vi "Steuerprogramm-04-02-17.vi"() -> ()   [LabVIEW 2010]
uses:
  Emil/Licor-Steuerung/HAGAR V/Licor-Steuerung/display/GUI_Cluster_sdv.ctl
  Emil/Licor-Steuerung/HAGAR V/Licor-Steuerung/display/GUI_Cluster_Parameter.ctl
  Emil/Licor-Steuerung/HAGAR V/Licor-Steuerung/control/Licor-Commands.ctl
  Emil/Licor-Steuerung/HAGAR V/Licor-Steuerung/control/Licor-Parameter.ctl
  Emil/Licor-Steuerung/LicorLI7000/conventions/Licor-Source.ctl
  Emil/Licor-Steuerung/HAGAR V/Licor-Steuerung/control/Licor-Pump.ctl
  Emil/Licor-Steuerung/HAGAR V/Licor-Steuerung/display/GUI_Cluster_Graph.ctl
  Emil/Licor-Steuerung/HAGAR V/Licor-Steuerung/control/Licor-Sequences.ctl
  <vilib>/rvi/interface/nirviMethod/nirviMethod.xnode
  C:/Users/HAGAR-IV/Desktop/Zeugs/markus/version feb 2012/FPGA Bitfiles/pertrasgcfpga2_FPGATarget_FPGA-Programm-01_A75D3647.lvbitx
  C:/Users/HAGAR-IV/Desktop/Zeugs/Johnny/pertrasgc fpga/FPGA-Programm-01-17.vi
  <vilib>/rvi/interface/common/niFpgaNodeNameForErrorReporting.ctl
  <vilib>/rvi/errors/niLvFpgaWhatHappensToTopLevelVI.ctl
  <vilib>/rvi/interface/nirviReadWriteControl/nirviReadWriteControl.xnode
  <vilib>/rvi/interface/nirviCloseFPGA/nirviCloseFPGA.xnode
  GVZwangs.vi
  GVProbenvol.vi
  GVZeitenZyklen.vi
  GVECDs.vi
  GVMethodenwechsel.vi
  GVTrapsMachs.vi
  GVHK1Hz.vi
  GVAIs.vi
  gvbooleschRT.vi
  GVMetavariablen.vi
  GVVentilposition.vi
  GVHorstSP.vi
  GVMWHorst.vi
  GVHeizenLH.vi
  <vilib>/Utility/error.llb/Error Cluster From Error Code.vi
  <vilib>/rvi/errors/niLvFpgaAdjustHostInterfaceError.vi
  GVaktuelleTDMS.vi
  Emil/Licor-Steuerung/HAGAR V/Licor-Steuerung/control/Emulate Licor output GV.vi
  GVChroms.vi
  GVZwangsMPV.vi
  <vilib>/FPGAPlugInAG/cRIO-9114/niLvFpga_Close_cRIO-9114.vi
  NiFpgaLv.dll
  Emil/Licor-Steuerung/HAGAR V/Licor-Steuerung/Licor-Steuerung.lvlib
  Emil/Licor-Steuerung/LicorLI7000/LicorLI7000.lvlib
panel:
  in  "Handbetrieb":bool
  in  "Methode speichern":bool
  out "ZyklusNummernGesamt":i32[](array[numeric])
  in  "veränderte Methode benutzen":bool
  in  "Methode verändern":bool
  out "ZyklusNummern":i32[](array[numeric])
  out "Big Ben, Methodenzeit, Zykluszeit0, Zykluszeit1, Zykluszeit2A, Zykluszeit2B":i32[](array[numeric])
  in  "global stop RT":bool
  in  "Methode":i32(ring) items=["Bedingsmethode", "Startmethode", "Meßmodus", "Shut-up-Methode", "Test", "HAG2 1/2", "Startmethode", "HAG2 1/2 Aufwärmen"]
  in  "Registerkarte":T1(tab)
  out "SHOK?":bool[](array[boolean])
  out "schnelle Heizungen":string[](array[string])
  out "schnelle Heizungen":dbl[](array[numeric])
  out "HorstOK?":bool[](array[boolean])
  out "AIs3OK?":bool[](array[boolean])
  out "AIs1OK?":bool[](array[boolean])
  out "AIs1":dbl[](array[numeric])
  out "AIs1":string[](array[string])
  out "AIs2":string[](array[string])
  out "AIs3":string[](array[string])
  out "AIs2":dbl[](array[numeric])
  out "AIs3":dbl[](array[numeric])
  out "Metavariablen":string[](array[string])
  out "Metavariablen":dbl[](array[numeric])
  out "MWHorst":dbl[](array[numeric])
  out "HorstRegler":string[](array[string])
  out "AIs2OK?":bool[](array[boolean])
  out "Ventilposition":i32=1 min=1 max=6 step=1
  out "MVOK?":bool[](array[boolean])
  in  "Color Box":u32(colorbox)
  out "Numeric":dbl
  out "Housekeeping1":cluster{dbl[], dbl[]}(graph)
  in  "Zeitachse1":i32(ring)=1 items=["Zykluszeit [s] Mod0", "Zykluszeit [s] Mod1", "Zykluszeit [s] Mod2A", "Zykluszeit [s] Mod2B"]
  in  "dargestellte Größe 1":i32(ring)=1 items=["T1-Trap1", "T1-Trap2", "T1-StirlingKühlkopf", "T1-PreCol1", "T1-PreCol2", "T1-MainCol1a", "T1-MainCol1b", "T1-MainCol2a", "T1-MainCol2b", "T1-Bronkhorst1a", "T1-Bronkhorst1b", "T1-Bronkhorst2a", "T1-Bronkhorst2b", "T1-2Pos1B", "T1-Spare9", "T1-2Pos1A", "T1-Spare10", "T1-TurboPump", "T1-StirlingPlatine", "T1-Spare5", "T1-Spare6", "T1-Spare7", "T1-Spare8", "F1-MFM1", "F1-MFM0D [mL]", "P1-MethaneHP", "P1-MethaneLP", "P1-Vacuum", "TurboSpeed", "I1-MS-AC", "I1-Trap1", "I1-Trap2", "T2-ECD1a", "T2-ECD1b", "T2-ECD2a", "T2-ECD2b", "T2-Col1a", "T2-Col1b", "T2-Col2a", "T2-Col2b", "T2-Spare1", "T2-Spare2", "T2-Oven_a", "T2-Oven_b", "T2-Spare3", "T2-Spare4", "T2-Spare5", "F2-MFM0", "F2-MFM2A", "F2-MFM2B", "P2-N2O_HP", "P2-N2O_LP", "P2-CO2_HP", "P2-CO2_LP", "AI-Spare1", "FL-MFM1000mL", "AI-Spare3", "AI-Spare4", "StirlingAlarm", "StirlingEmerg.", "AI-Spare7", "AI-Spare8", "AI-Spare9", "FL-MFM30mL", "T0-DC/DC5", "I0-24V_M0", "I0-48V_M1", "I0-24V_M1", "I0-28V_M2", "T0-Spare3", "T0-Spare2", "T0-Spare4", "T0-DC/DC7", "I0-20V_Laptop", "I0-28V_M1", "I0-24V_M2", "I0-12V_Licor", "T0-Spare1", "T0-Drier", "T0-Spare5", "F0-MFM0A [L]", "TL-Licor_a", "P0-Span-HP", "P0-spare1", "P0-Stickstoff-LP", "P0-Helium-LP", "P0-Cal-HP", "P0-P9Tavco[bar]", "F0-MFM0B [L]", "TL-Licor_b", "P0-Span-LP", "P0-spare2", "P0-Stickstoff-HP", "P0-Helium-HP", "P0-Cal-LP", "F0-MFM3", "TemperaturTrap1[°C]", "TemperaturTrap2[°C]", "TemperaturPreMach1[°C]", "TemperaturPreMach2[°C]", "TemperaturMainMach1[°C]", "TemperaturMainMach2[°C]", "PrC0", "PrC0-Licor", "PrC1-Säule2", "PrC1-Säule1", "MFC1-Sample", "MFC1-Methan", "PrC1-BackFlush1", "PrC1-BackFlush2", "MFC2A", "MFC2B", "MFC2C", "PrC2A", "MFC2D", "MFC2E", "PrC2B"]
  out "Housekeeping2":cluster{dbl[], dbl[]}(graph)
  in  "Zeitachse2":i32(ring)=1 items=["Zykluszeit [s] Mod0", "Zykluszeit [s] Mod1", "Zykluszeit [s] Mod2A", "Zykluszeit [s] Mod2B"]
  in  "dargestellte Größe 2":i32(ring)=1 items=["T1-Trap1", "T1-Trap2", "T1-StirlingKühlkopf", "T1-PreCol1", "T1-PreCol2", "T1-MainCol1a", "T1-MainCol1b", "T1-MainCol2a", "T1-MainCol2b", "T1-Bronkhorst1a", "T1-Bronkhorst1b", "T1-Bronkhorst2a", "T1-Bronkhorst2b", "T1-2Pos1B", "T1-Spare9", "T1-2Pos1A", "T1-Spare10", "T1-TurboPump", "T1-StirlingPlatine", "T1-Spare5", "T1-Spare6", "T1-Spare7", "T1-Spare8", "F1-MFM1", "F1-MFM0D [mL]", "P1-MethaneHP", "P1-MethaneLP", "P1-Vacuum", "TurboSpeed", "I1-MS-AC", "I1-Trap1", "I1-Trap2", "T2-ECD1a", "T2-ECD1b", "T2-ECD2a", "T2-ECD2b", "T2-Col1a", "T2-Col1b", "T2-Col2a", "T2-Col2b", "T2-Spare1", "T2-Spare2", "T2-Oven_a", "T2-Oven_b", "T2-Spare3", "T2-Spare4", "T2-Spare5", "F2-MFM0", "F2-MFM2A", "F2-MFM2B", "P2-N2O_HP", "P2-N2O_LP", "P2-CO2_HP", "P2-CO2_LP", "AI-Spare1", "FL-MFM1000mL", "AI-Spare3", "AI-Spare4", "StirlingAlarm", "StirlingEmerg.", "AI-Spare7", "AI-Spare8", "AI-Spare9", "FL-MFM30mL", "T0-DC/DC5", "I0-24V_M0", "I0-48V_M1", "I0-24V_M1", "I0-28V_M2", "T0-Spare3", "T0-Spare2", "T0-Spare4", "T0-DC/DC7", "I0-20V_Laptop", "I0-28V_M1", "I0-24V_M2", "I0-12V_Licor", "T0-Spare1", "T0-Drier", "T0-Spare5", "F0-MFM0A [L]", "TL-Licor_a", "P0-Span-HP", "P0-spare1", "P0-Stickstoff-LP", "P0-Helium-LP", "P0-Cal-HP", "P0-P9Tavco[bar]", "F0-MFM0B [L]", "TL-Licor_b", "P0-Span-LP", "P0-spare2", "P0-Stickstoff-HP", "P0-Helium-HP", "P0-Cal-LP", "F0-MFM3", "TemperaturTrap1[°C]", "TemperaturTrap2[°C]", "TemperaturPreMach1[°C]", "TemperaturPreMach2[°C]", "TemperaturMainMach1[°C]", "TemperaturMainMach2[°C]", "PrC0", "PrC0-Licor", "PrC1-Säule2", "PrC1-Säule1", "MFC1-Sample", "MFC1-Methan", "PrC1-BackFlush1", "PrC1-BackFlush2", "MFC2A", "MFC2B", "MFC2C", "PrC2A", "MFC2D", "MFC2E", "PrC2B"]
  out "Detektor 2":cluster{dbl[], dbl[]}[](graph)
  in  "Detektor":i32(ring) items=["ECD1", "ECD2"]
  in  "HK1YMin":dbl
  in  "HK1YMax":dbl=100.0
  in  "HK2YMin":dbl
  in  "HK2YMax":dbl=100.0
  in  "DetYMin":dbl
  in  "DetYMax":dbl=100.0
  out "schnelleAnzeige":cluster{dbl[], dbl[]}(graph)
  in  "TafelWischen!":bool
  in  "dargestellte Größe 3":i32(ring)=1 items=["TemperaturTrap1[°C]", "TemperaturTrap2[°C]", "TemperaturPreMach1[°C]", "TemperaturPreMach2[°C]", "TemperaturMainMach1[°C]", "TemperaturMainMach2[°C]", "PrC0", "PrC0-Licor", "PrC1-Säule2", "PrC1-Säule1", "MFC1-Sample", "MFC1-Methan", "PrC1-BackFlush1", "PrC1-BackFlush2", "MFC2A", "MFC2B", "MFC2C", "PrC2A", "MFC2D", "MFC2E", "PrC2B"]
  in  "An/Aus":bool
  in  "Registerkarte 2":T2(tab)
  in  "GUI_Cluster_Graph":T3={"time (global)"=0.0, "command queue"=[], "Rohdaten"=[], "Graph"={"X"=[], "Y"=[]}, "Manuelle Steuerung"={"Sequenz"=enum."test", "Manuelle Steuerung An/Aus"=FALSE}, "Sequenz out"={"sequence"=enum."WAIT", "Zeitpunkt next"=0.0, "delta t"=0.0}} caption="Cluster" {"Sequenz out"."Zeitpunkt next" format="%<%H:%M:%S%3u>T"; "time (global)" format="%<%H:%M:%S%3u\n%m/%d/%y>T"}
  in  "GUI_Cluster_Parameter":T5={"warmup (sequence)"=[{"time"=60, "Enum"=enum."wait"}], "calibrate S (sequence)"=[{"time"=60, "Enum"=enum."wait"}, {"time"=2, "Enum"=enum."getCalibrationParameter"}, {"time"=8, "Enum"=enum."calibration-S-CO2"}, {"time"=2, "Enum"=enum."getCalibrationParameter"}], "calibrate Z (sequence)"=[{"time"=60, "Enum"=enum."wait"}, {"time"=2, "Enum"=enum."getCalibrationParameter"}, {"time"=8, "Enum"=enum."calibration-Z-H2O"}, {"time"=2, "Enum"=enum."getCalibrationParameter"}, {"time"=8, "Enum"=enum."calibration-Z-CO2"}, {"time"=2, "Enum"=enum."getCalibrationParameter"}], "initialize (sequence)"=[{"time"=30, "Enum"=enum."wait"}, {"time"=2, "Enum"=enum."setPumpSlow"}, {"time"=2, "Enum"=enum."setPumpMedium"}, {"time"=2, "Enum"=enum."setPumpFast"}, {"time"=10, "Enum"=enum."initialize"}, {"time"=4, "Enum"=enum."getCalibrationParameter"}, {"time"=2, "Enum"=enum."resetH2O"}, {"time"=4, "Enum"=enum."resetCO2"}, {"time"=4, "Enum"=enum."getCalibrationParameter"}, {"time"=2, "Enum"=enum."setZeroParameter"}, {"time"=4, "Enum"=enum."getCalibrationParameter"}, {"time"=2, "Enum"=enum."setReference"}, {"time"=4, "Enum"=enum."getLicorTime"}, {"time"=5, "Enum"=enum."getInfo"}], "Licor-parameter"={"CO2 ref"=402.3, "CO2 span"=392.3, "H2O ref"=0.0, "H2O span"=0.0, "Zi"=1.2, "Zt"=6.494e-05, "Zm"=0.0, "S"=1.34, "Temp [C]"=45.0, "Pressure [hPa]"=1013.0, "Licor-Sources"=["CO2A W", "CO2B W", "H2OA W", "H2OB W", "T C", "T V", "P kPa", "P V", "RH %", "CO2A um/m", "CO2B um/m", "H2OA mm/m", "H2OB mm/m"], "Licor-Pump"="Off", "Zeitstempel"=timestamp(0 s since 1904-01-01)}} {"Licor-parameter"."Pressure [hPa]" format="%_5g"; "Licor-parameter"."Temp [C]" format="%.2f"; "Licor-parameter"."CO2 ref" format="%.2f"; "Licor-parameter"."CO2 span" format="%.2g"; "Licor-parameter"."H2O ref" format="%.2g"; "Licor-parameter"."H2O span" format="%.2g"; "Licor-parameter"."Zt" format="%#_4g"}
  in  "GUI_Cluster_sdv":T10={"Graph_sdv"={"X"=[], "Y"=[]}, "Breite"=20, "Berechnen"=FALSE, "residue"=0.0} {"residue" format="%_6g"}
  in  "VISA resource name":refnum<visa-resource-name>="ASRL1::INSTR" caption="VISA-Ressourcenname"
  in  "ServosWarmHigh (us)KaltHigh(us)":T11={"Servo1WarmHigh(us)"=1000, "Servo1KaltHigh(us)"=1000, "Servo2WarmHigh(us)"=2030, "Servo2KaltHigh(us)"=2030}
  out "TDMSwriteECD":errorcluster
  out "AIsFIFOread":errorcluster
  out "MWTrapsMachs":errorcluster
  out "TDMSwriteHK":errorcluster
  out "TDMScloseHK":errorcluster
  out "TDMSopenHK":errorcluster
  out "TDMScloseECD2":errorcluster
  out "TDMSopenECD2":errorcluster
  out "TDMScloseECD1":errorcluster
  out "TDMSopenECD1":errorcluster
  out "FIFOwriteRS485":errorcluster
  out "SerielleKomm.":errorcluster
  out "LH":errorcluster
  out "Zyklus":errorcluster
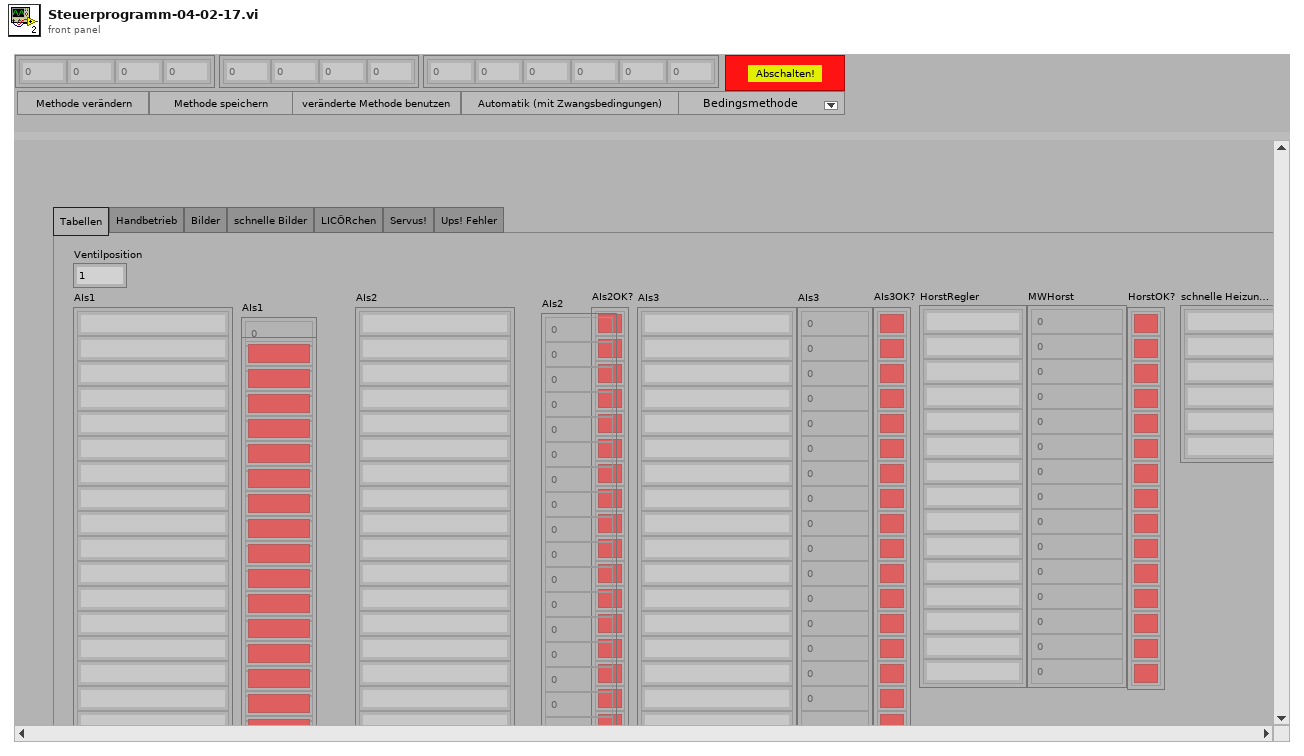
[diagram p1: front panel]
types:
  T1 = enum32{"Tabellen", "Handbetrieb", "Bilder", "schnelle Bilder", "LICÖRchen", "Servus!", "Ups! Fehler"}
  T2 = enum32{"Graph", "Parameter / Sequenzen", "sdv", "debug"}
  T3 = typedef "Licor-Steuerung.lvlib/GUI_Cluster_Graph.ctl" = cluster{"time (global)":dbl, "command queue":cluster{"Zeit [s]":i32, "Befehl":string}[], "Rohdaten":string[], "Graph":cluster{"X":dbl[], "Y":dbl[]}, "Manuelle Steuerung":cluster{"Sequenz":T4, "Manuelle Steuerung An/Aus":bool}, "Sequenz out":cluster{"sequence":T4, "Zeitpunkt next":dbl, "delta t":dbl}}
  T4 = typedef "Licor-Steuerung.lvlib/Licor-Sequences.ctl" = enum16{"test", "WAIT", "warmup", "initialize", "calibrate Z", "calibrate S"}
  T5 = typedef "Licor-Steuerung.lvlib/GUI_Cluster_Parameter.ctl" = cluster{"warmup (sequence)":cluster{"time":i32, "Enum":T6}[], "calibrate S (sequence)":cluster{"time":i32, "Enum":T6}[], "calibrate Z (sequence)":cluster{"time":i32, "Enum":T6}[], "initialize (sequence)":cluster{"time":i32, "Enum":T6}[], "Licor-parameter":T7}
  T6 = typedef "Licor-Steuerung.lvlib/Licor-Commands.ctl" = enum16{"wait", "initialize", "resetCO2", "resetH2O", "getReference", "setReference", "calibration-Z-CO2", "calibration-Z-H2O", "calibration-S-CO2", "calibration-S-H2O", "getCalibrationParameter", "setZeroParameter", "setLicorTime", "getLicorTime", "setPumpFlowrate", "setPumpSlow", "setPumpMedium", "setPumpFast", "getInfo"}
  T7 = typedef "Licor-Steuerung.lvlib/Licor-Parameter.ctl" = cluster{"CO2 ref":dbl, "CO2 span":dbl, "H2O ref":dbl, "H2O span":dbl, "Zi":dbl, "Zt":dbl, "Zm":dbl, "S":dbl, "Temp [C]":dbl, "Pressure [hPa]":dbl, "Licor-Sources":T8[], "Licor-Pump":T9, "Zeitstempel":timestamp}
  T8 = typedef "LicorLI7000.lvlib/Licor-Source.ctl" = string
  T9 = typedef "Licor-Steuerung.lvlib/Licor-Pump.ctl" = string
  T10 = typedef "Licor-Steuerung.lvlib/GUI_Cluster_sdv.ctl" = cluster{"Graph_sdv":cluster{"X":dbl[], "Y":dbl[]}, "Breite":i32, "Berechnen":bool, "residue":dbl}
  T11 = cluster{"Servo1WarmHigh(us)":u32, "Servo1KaltHigh(us)":u32, "Servo2WarmHigh(us)":u32, "Servo2KaltHigh(us)":u32}
  T12 = cluster{"DIOsMod0Nr":i32[], "DIOsMod1Nr":i32[], "DIOsMod2ANr":i32[], "DIOsMod2BNr":i32[], "AIsLH":i32[], "AnzahlRegler/Modul":i32[], "Regler für den Probenfluß":i32, "SPvorgebenMod0":string[], "SPvorgebenMod1":string[], "SPvorgebenMod2A":string[], "SPvorgebenMod2B":string[], "MWAntwortMod0":string[], "MWAntwortMod1":string[], "MWAntwortMod2A":string[], "MWAntwortMod2B":string[], "FaktorMod0":dbl[], "FaktorMod1":dbl[], "FaktorMod2A":dbl[], "FaktorMod2B":dbl[], "MWabfragenMod0":string[], "MWabfragenMod1":string[], "MWabfragenMod2A":string[], "MWabfragenMod2B":string[], "Modul1/AI koeff":dbl[][], "Modul2/AI koeff":dbl[][], "Modul3/AI koeff":dbl[][], "Traps/MachsKoeff":dbl[][], "Modul1/AIsNamen":string[], "Modul2/AIsNamen":string[], "Modul3/AIsNamen":string[], "DIOsMod0Name":string[], "DIOsMod1Name":string[], "DIOsMod2AName":string[], "DIOsMod2BName":string[], "ReglerNameMod0":string[], "ReglerNameMod1":string[], "ReglerNameMod2A":string[], "ReglerNameMod2B":string[], "Startmethode":i32, "Dateiordner Housekeeping":path, "Dateiname Housekeeping":string, "DateiordnerECD1":path, "DateinameECD1":string, "DateiordnerECD2":path, "DateinameECD2":string, "LangsameHeizungen":string[], "ModuleLH":i32[], "Metavariablen":string[], "Modul1/AI sicherer Bereich":dbl[][], "Modul2/AI sicherer Bereich":dbl[][], "Modul3/AI sicherer Bereich":dbl[][], "Traps/Machs sicherer Bereich":dbl[][], "ReglerMod0 sicherer Bereich":dbl[][], "ReglerMod1 sicherer Bereich":dbl[][], "ReglerMod2A sicherer Bereich":dbl[][], "ReglerMod2B sicherer Bereich":dbl[][], "Metavariablen grüner Bereich":dbl[][]}
  T13 = cluster{"Zykluslängen [s]":dbl[], "ZeitpktDIOsMod0":dbl[], "ZeitpktDIOsMod1":dbl[], "ZeitpktDIOsMod2A":dbl[], "ZeitpktDIOsMod2B":dbl[], "DIOsSPMod0":bool[][], "DIOsSPMod1":bool[][], "DIOsSPMod2A":bool[][], "DIOsSPMod2B":bool[][], "Mod0HorstZeitpkt":dbl[], "Mod1HorstZeitpkt":dbl[], "Mod2AHorstZeitpkt":dbl[], "Mod2BHorstZeitpkt":dbl[], "HorstSPMod0":dbl[][], "HorstSPMod1":dbl[][], "HorstSPMod2A":dbl[][], "HorstSPMod2B":dbl[][], "LHSetpoints":dbl[], "LHHeizen?":bool[], "ZPktFPGABoolesch":dbl[], "FPGABoolesch":bool[][], "ZeitpktFPGAPID":dbl[], "FPGAPID":cluster{"proportional gain (Kc)":fxp<+/-,16,8>, "integral gain (Kc*Ts/Ti)":fxp<+/-,16,8>, "derivative gain (Kc*Td/Ts)":fxp<+/-,16,8>}[][], "ZeitpktFPGAFixp":dbl[], "SHSetpoints":dbl[][], "t_PreMach1":dbl[], "T_PreMach1":dbl[], "t_PreMach2":dbl[], "T_PreMach2":dbl[], "PIDs für \"träge\" Heizungen":cluster{"proportional gain (Kc)":dbl, "integral time (Ti, min)":dbl, "derivative time (Td, min)":dbl}[], "Zwangsbedingungen":dbl[][], "Dateien fürs MS schicken?":bool, "ZeitpunkteMPV":dbl[], "SPMPV":i32[], "ZeitpktMS-1":dbl, "ZeitpktMS-2":dbl, "Int.Start1":dbl, "Int.Stop1":dbl, "Int.Start2":dbl, "Int.Stop2":dbl, "Methodenname":string, "t_MainMach1":dbl[], "T_MainMach1":dbl[], "t_MainMach2":dbl[], "T_MainMach2":dbl[]}[]
  T14 = enum16{"open", "replace", "create", "open or create", "replace or create", "replace or create with confirmation"}
  T15 = typedef "niFpgaNodeNameForErrorReporting.ctl" = enum16{"Open FPGA VI Reference", "Read/Write Control", "Invoke Method: Abort", "Invoke Method: Acknowledge IRQ", "Invoke Method: Download", "Invoke Method: FIFO.Configure", "Invoke Method: FIFO.Read", "Invoke Method: FIFO.Start", "Invoke Method: FIFO.Stop", "Invoke Method: FIFO.Write", "Invoke Method: Reset", "Invoke Method: Run", "Invoke Method: Wait on IRQ", "Close FPGA VI Reference"}
  T16 = typedef "niLvFpgaWhatHappensToTopLevelVI.ctl" = enum16{"top level VI scripted behind XNode", "top level VI inlined behind XNode"}
  T17 = cluster{"Zyklus1":i32, "Zeitachse1":i32, "dargestellte Größe 1":i32, "Zyklus2":i32, "Zeitachse2":i32, "dargestellte Größe 2":i32}
  T18 = cluster{"Modul1/AI sicherer Bereich":dbl[][], "Modul2/AI sicherer Bereich":dbl[][], "Modul3/AI sicherer Bereich":dbl[][], "Traps/Machs sicherer Bereich":dbl[][], dbl[][], "Metavariablen grüner Bereich":dbl[][]}
  T19 = cluster{"DIOsMod0Name":string[], "DIOsMod1Name":string[], "DIOsMod2AName":string[], "DIOsMod2BName":string[], "ReglerNameMod0":string[], "ReglerNameMod1":string[], "ReglerNameMod2A":string[], "ReglerNameMod2B":string[], "LangsameHeizungen":string[]}
  T20 = cluster{"Zykluslängen [s]":dbl[], "ZeitpktDIOsMod0":dbl[], "ZeitpktDIOsMod1":dbl[], "ZeitpktDIOsMod2A":dbl[], "ZeitpktDIOsMod2B":dbl[], "DIOsSPMod0":bool[][], "DIOsSPMod1":bool[][], "DIOsSPMod2A":bool[][], "DIOsSPMod2B":bool[][], "Mod0HorstZeitpkt":dbl[], "Mod1HorstZeitpkt":dbl[], "Mod2AHorstZeitpkt":dbl[], "Mod2BHorstZeitpkt":dbl[], "HorstSPMod0":dbl[][], "HorstSPMod1":dbl[][], "HorstSPMod2A":dbl[][], "HorstSPMod2B":dbl[][], "LHSetpoints":dbl[], "LHHeizen?":bool[], "ZPktFPGABoolesch":dbl[], "FPGABoolesch":bool[][], "ZeitpktFPGAPID":dbl[], "FPGAPID":cluster{"proportional gain (Kc)":fxp<+/-,16,8>, "integral gain (Kc*Ts/Ti)":fxp<+/-,16,8>, "derivative gain (Kc*Td/Ts)":fxp<+/-,16,8>}[][], "ZeitpktFPGAFixp":dbl[], "SHSetpoints":dbl[][], "t_PreMach1":dbl[], "T_PreMach1":dbl[], "t_PreMach2":dbl[], "T_PreMach2":dbl[], "PIDs für \"träge\" Heizungen":cluster{"proportional gain (Kc)":dbl, "integral time (Ti, min)":dbl, "derivative time (Td, min)":dbl}[], "Zwangsbedingungen":dbl[][], "Dateien fürs MS schicken?":bool, "ZeitpunkteMPV":dbl[], "SPMPV":i32[], "ZeitpktMS-1":dbl, "ZeitpktMS-2":dbl, "Int.Start1":dbl, "Int.Stop1":dbl, "Int.Start2":dbl, "Int.Stop2":dbl, "Methodenname":string, "t_MainMach1":dbl[], "T_MainMach1":dbl[], "t_MainMach2":dbl[], "T_MainMach2":dbl[]}
  T21 = cluster{"created path":path, "created path":path, "created path":path, "Dateiname Housekeeping":string, "DateinameECD1":string, "DateinameECD2":string, "tdms0":refnum<k34>, "tdms1":refnum<k34>, "tdms0":refnum<k34>, "tdms1":refnum<k34>, "tdms0":refnum<k34>, "tdms1":refnum<k34>}
  T22 = cluster{"proportional gain (Kc)":fxp<+/-,16,8>, "integral gain (Kc*Ts/Ti)":fxp<+/-,16,8>, "derivative gain (Kc*Td/Ts)":fxp<+/-,16,8>}[][]
  T23 = cluster{"proportional gain (Kc)":dbl, "integral time (Ti, min)":dbl, "derivative time (Td, min)":dbl}[]
  T24 = cluster{cluster{"ZeitpktDIOsMod2B":dbl[]}[], cluster{"DIOsSPMod2B":bool[][]}[], cluster{"Mod2BHorstZeitpkt":dbl[]}[], cluster{"HorstSPMod2B":dbl[][]}[], "LHHeizen?":bool[], "ZPktFPGABoolesch":dbl[], "FPGABoolesch":bool[][], "ZeitpktFPGAPID":dbl[], "FPGAPID":cluster{"proportional gain (Kc)":fxp<+/-,16,8>, "integral gain (Kc*Ts/Ti)":fxp<+/-,16,8>, "derivative gain (Kc*Td/Ts)":fxp<+/-,16,8>}[][], "ZeitpktFPGAFixp":dbl[], "SHSetpoints":dbl[][], "t_PreMach1":dbl[], "T_PreMach1":dbl[], "t_PreMach2":dbl[], "T_PreMach2":dbl[], "ZeitpunkteMPV":dbl[], "SPMPV":i32[], "t_MainMach1":dbl[], "T_MainMach1":dbl[], "t_MainMach2":dbl[], "T_MainMach2":dbl[]}
  T25 = cluster{"Zykluslängen [s]":dbl[], "ZeitpktDIOsMod0":dbl[], "ZeitpktDIOsMod1":dbl[], "ZeitpktDIOsMod2A":dbl[], "ZeitpktDIOsMod2B":dbl[], "DIOsSPMod0":bool[][], "DIOsSPMod1":bool[][], "DIOsSPMod2A":bool[][], "DIOsSPMod2B":bool[][], "Mod0HorstZeitpkt":dbl[], "Mod1HorstZeitpkt":dbl[], "Mod2AHorstZeitpkt":dbl[], "Mod2BHorstZeitpkt":dbl[], "HorstSPMod0":dbl[][], "HorstSPMod1":dbl[][], "HorstSPMod2A":dbl[][], "HorstSPMod2B":dbl[][], "LangsameHeizungenSP":dbl[], "LHHeizen?":bool[], "ZPktFPGABoolesch":dbl[], "FPGABoolesch":bool[][], "ZeitpktFPGAPID":dbl[], "FPGAPID":cluster{"proportional gain (Kc)":fxp<+/-,16,8>, "integral gain (Kc*Ts/Ti)":fxp<+/-,16,8>, "derivative gain (Kc*Td/Ts)":fxp<+/-,16,8>}[][], "ZeitpktFPGAFixp":dbl[], "FPGAFixp":dbl[][], "t_PreMach1":dbl[], "T_PreMach1":dbl[], "t_PreMach2":dbl[], "T_PreMach2":dbl[], "PIDs für \"träge\" Heizungen":cluster{"proportional gain (Kc)":dbl, "integral time (Ti, min)":dbl, "derivative time (Td, min)":dbl}[], "Zwangsbedingungen":dbl[][], "MS-Daten?":bool, "ZeitpunkteMPV":dbl[], "SetpointMPV":i32[], "ZeitpktMS-1":dbl, "ZeitpktMS-2":dbl, "Int.Start1":dbl, "Int.Stop1":dbl, "Int.Start2":dbl, "Int.Stop2":dbl, "Methodenname":string, "t_MainMach1":dbl[], "T_MainMach1":dbl[], "t_MainMach2":dbl[], "T_MainMach2":dbl[]}
  T26 = cluster{"ZyklusNummern":i32[], "ZeilennummernDIOs":i32[], "ZwangsDIO?":cluster{bool[]}[], "ZeilennummernHorst":i32[], "ZwangsHorst?":cluster{bool[]}[], "ZeileFPGABoolesch":i32, "ZwangsFPGABoolesch?":bool[], "ZeileFPGAPID":i32, "ZeileFPGAFixp":i32, "ZeilePreMach1":i32, "ZeilePreMach2":i32, "ZeilennummerMPV":i32, "ZeileMainMach1":i32, "ZeileMainMach2":i32, "ZwangsMPV?":bool}
  T27 = cluster{"ZyklusNummern":i32[], i32[], "ZwangsDIO?":cluster{bool[]}[], i32[], "ZwangsHorst?":cluster{bool[]}[], i32, "ZwangsFPGABoolesch?":bool[], i32, i32, "ZeileMach":i32, "ZeileMach":i32, i32, "ZeileMach":i32, "ZeileMach":i32, "ZwangsMPV?":bool}
  T28 = cluster{string[], string[], string[], dbl[], dbl[], dbl[]}
  T29 = cluster{"Befehle1":string[], "Befehle2":string[], "Befehle3":string[]}
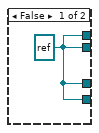
[diagram p2: hidden frame]
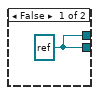
[diagram p3: hidden frame]
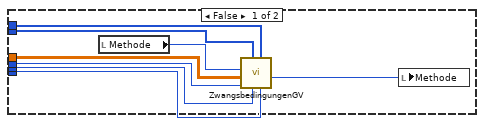
[diagram p11: hidden frame]
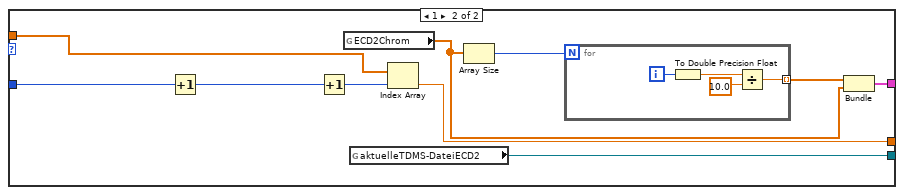
[diagram p13: hidden frame]
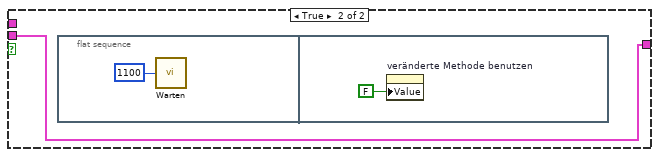
[diagram p14: hidden frame]
diagram:
  n1 = Open/Create/Replace File(file path (use dialog)=path "c:/einstellungen.perx" ("Datei (Dialog verwenden)"), operation (0:open)=T14."open" ("Operation (0:Öffnen)")) -> (refnum out=w13:refnum<file>)  [unwired: 4 in, 2 out]
  n2 = Open/Create/Replace File(file path (use dialog)=path "c:/methoden.perx" ("Datei (Dialog verwenden)"), operation (0:open)=T14."open" ("Operation (0:Öffnen)")) -> (refnum out=w8:refnum<file>)  [unwired: 4 in, 2 out]
  n3 = Read from Binary File(5:T12 {"DIOsMod0Nr"=[], "DIOsMod1Nr"=[], "DIOsMod2ANr"=[], "DIOsMod2BNr"=[], "AIsLH"=[], "AnzahlRegler/Modul"=[], "Regler für den Probenfluß"=0, "SPvorgebenMod0"=[], "SPvorgebenMod1"=[], "SPvorgebenMod2A"=[], "SPvorgebenMod2B"=[], "MWAntwortMod0"=[], "MWAntwortMod1"=[], "MWAntwortMod2A"=[], "MWAntwortMod2B"=[], "FaktorMod0"=[], "FaktorMod1"=[], "FaktorMod2A"=[], "FaktorMod2B"=[], "MWabfragenMod0"=[], "MWabfragenMod1"=[], "MWabfragenMod2A"=[], "MWabfragenMod2B"=[], "Modul1/AI koeff"=[], "Modul2/AI koeff"=[], "Modul3/AI koeff"=[], "Traps/MachsKoeff"=[], "Modul1/AIsNamen"=[], "Modul2/AIsNamen"=[], "Modul3/AIsNamen"=[], "DIOsMod0Name"=[], "DIOsMod1Name"=[], "DIOsMod2AName"=[], "DIOsMod2BName"=[], "ReglerNameMod0"=[], "ReglerNameMod1"=[], "ReglerNameMod2A"=[], "ReglerNameMod2B"=[], "Startmethode"=0, "Dateiordner Housekeeping"=path "", "Dateiname Housekeeping"="", "DateiordnerECD1"=path "", "DateinameECD1"="", "DateiordnerECD2"=path "", "DateinameECD2"="", "LangsameHeizungen"=[], "ModuleLH"=[], "Metavariablen"=[], "Modul1/AI sicherer Bereich"=[], "Modul2/AI sicherer Bereich"=[], "Modul3/AI sicherer Bereich"=[], "Traps/Machs sicherer Bereich"=[], "ReglerMod0 sicherer Bereich"=[], "ReglerMod1 sicherer Bereich"=[], "ReglerMod2A sicherer Bereich"=[], "ReglerMod2B sicherer Bereich"=[], "Metavariablen grüner Bereich"=[]} ("output cluster"), 11:w13) -> (2:w11:T12, 3:w12:refnum<file>)  [unwired: 4 in, 2 out]
  n4 = Read from Binary File(5:T13 [], 11:w8) -> (2:w6:T13, 3:w7:refnum<file>)  [unwired: 4 in, 2 out]
  n5 = Close File(refnum=w12) -> ()  [unwired: 1 in, 2 out]
  n6 = Close File(refnum=w7) -> ()  [unwired: 1 in, 2 out]
  n7 = flat-sequence {
    tunnel: [w65] -> w41
    tunnel: [w122] -> w40
    tunnel: [w69] -> w38
    tunnel: [w254] -> w37
    tunnel: [w256] -> w36
    tunnel: [w248] -> w35
    tunnel: [w255] -> w34
    tunnel: [w178] -> w33
    tunnel: [w247] -> w32
    tunnel: [w246] -> w31
    tunnel: [w240] -> w30
    tunnel: [w181] -> w29
    tunnel: [w155] -> w28
    tunnel: [w253] -> w27
    tunnel: [w245] -> w26
    tunnel: [w244] -> w25
    tunnel: [w236] -> w24
    tunnel: [w235] -> w23
    tunnel: [w234] -> w22
    tunnel: [w233] -> w21
    tunnel: [w232] -> w20
    tunnel: [w231] -> w19
    tunnel: [w228] -> w18
    tunnel: [w210] -> w17
    tunnel: w11 -> [w98]
    tunnel: [w209] -> w16
    tunnel: w6 -> [w123]
    tunnel: [w122] -> w5
    tunnel: [w98] -> w3
    tunnel: [w60] -> w1
    tunnel: w41 -> [w453]
    tunnel: w40 -> [w526]
    tunnel: [w453] -> w39
    tunnel: w38 -> [_]
    tunnel: w37 -> [w484]
    tunnel: w36 -> [w483]
    tunnel: w35 -> [w485]
    tunnel: w34 -> [w482]
    tunnel: w33 -> [w457]
    tunnel: w32 -> [w452]
    tunnel: w31 -> [w449]
    tunnel: w30 -> [w446]
    tunnel: w29 -> [w447]
    tunnel: w28 -> [w450]
    tunnel: w27 -> [w524]
    tunnel: w26 -> [w455]
    tunnel: w25 -> [w525]
    tunnel: w24 -> [w428]
    tunnel: w23 -> [w427]
    tunnel: w22 -> [w426]
    tunnel: w21 -> [w522]
    tunnel: w20 -> [w521]
    tunnel: w19 -> [w520]
    tunnel: w18 -> [w474]
    tunnel: w17 -> [w456]
    tunnel: w16 -> [w445]
    tunnel: w6 -> [w444]
    tunnel: w5 -> [w442]
    tunnel: w3 -> [_]
    tunnel: w1 -> [w421]
    tunnel: w39 -> [w1351]
    frame #0 {
      w124 = TRUE
      w139 = 0.0 ("Probenvol.1")
      w146 = dbl[] [-1.0] ("ECD1MW")
      w147 = FALSE ("ECD1Empfangen?")
      w138 = string[] ["TemperaturTrap1[°C]", "TemperaturTrap2[°C]", "TemperaturPreMach1[°C]", "TemperaturPreMach2[°C]", "TemperaturMainMach1[°C]", "TemperaturMainMach2[°C]"]
      w251 = string[] ["Big Ben [s]", "Methodenzeit [s]", "Zykluszeit [s] Mod0", "Zykluszeit [s] Mod1", "Zykluszeit [s] Mod2A", "Zykluszeit [s] Mod2B"]
      w241 = FALSE ("Undefinierte Werte möglich")
      w242 = FALSE ("global stop RT")
      n8 = for {
        tunnel: [w416] -> w249 mode=indexing
        tunnel: w123 -> [w417] mode=indexing
        n9 = Unbundle(w417) -> ("Methodenname"=w416:string)  [unwired: 44 out]
      }
      n10 = call "FPGA-Start-01-17.vi"() -> ("error out"=w69:errorcluster, "FPGA VI Reference Out"=w68:refnum<k20>)  [unwired: 2 in]
      n11 = Unbundle(w98) -> ("DIOsMod0Nr"=w165:i32[], "DIOsMod1Nr"=w164:i32[], "DIOsMod2ANr"=w163:i32[], "DIOsMod2BNr"=w162:i32[], "AIsLH"=w152:i32[], "AnzahlRegler/Modul"=w155:i32[], "Regler für den Probenfluß"=w209:i32, "SPvorgebenMod0"=w208:string[], "SPvorgebenMod1"=w207:string[], "SPvorgebenMod2A"=w206:string[], "SPvorgebenMod2B"=w205:string[], "MWAntwortMod0"=w204:string[], "MWAntwortMod1"=w203:string[], "MWAntwortMod2A"=w202:string[], "MWAntwortMod2B"=w201:string[], "FaktorMod0"=w200:dbl[], "FaktorMod1"=w199:dbl[], "FaktorMod2A"=w198:dbl[], "FaktorMod2B"=w197:dbl[], "MWabfragenMod0"=w196:string[], "MWabfragenMod1"=w195:string[], "MWabfragenMod2A"=w194:string[], "MWabfragenMod2B"=w193:string[], "Modul1/AI koeff"=w192:dbl[][], "Modul2/AI koeff"=w191:dbl[][], "Modul3/AI koeff"=w190:dbl[][], "Traps/MachsKoeff"=w189:dbl[][], "Modul1/AIsNamen"=w188:string[], "Modul2/AIsNamen"=w187:string[], "Modul3/AIsNamen"=w186:string[], "DIOsMod0Name"=w96:string[], "DIOsMod1Name"=w97:string[], "DIOsMod2AName"=w95:string[], "DIOsMod2BName"=w94:string[], "ReglerNameMod0"=w113:string[], "ReglerNameMod1"=w112:string[], "ReglerNameMod2A"=w111:string[], "ReglerNameMod2B"=w110:string[], "Startmethode"=w122:i32, "Dateiordner Housekeeping"=w93:path, "Dateiname Housekeeping"=w185:string, "DateiordnerECD1"=w107:path, "DateinameECD1"=w184:string, "DateiordnerECD2"=w106:path, "DateinameECD2"=w183:string, "LangsameHeizungen"=w182:string[], "ModuleLH"=w177:i32[], "Metavariablen"=w117:string[], "Modul1/AI sicherer Bereich"=w64:dbl[][], "Modul2/AI sicherer Bereich"=w63:dbl[][], "Modul3/AI sicherer Bereich"=w62:dbl[][], "Traps/Machs sicherer Bereich"=w61:dbl[][], "ReglerMod0 sicherer Bereich"=w59:dbl[][], "ReglerMod1 sicherer Bereich"=w58:dbl[][], "ReglerMod2A sicherer Bereich"=w57:dbl[][], "ReglerMod2B sicherer Bereich"=w56:dbl[][], "Metavariablen grüner Bereich"=w54:dbl[][])
      "Metavariablen" <- w117
      n12 = Initialize Array(0, 4 ("Dimension")) -> (w140:i32[])
      n13 = Initialize Array(0.0 ("Element"), 6 ("Dimension")) -> (w143:dbl[])
      n14 = global write "GVMethodenwechsel.vi" "Methodenwechsel?"(FALSE ("Methodenwechsel?")) -> ()
      n15 = Build Array (concatenate)(w59, w58, w57, w56) -> (w55:dbl[][])
      n16 = Bundle("Modul1/AI sicherer Bereich"=w64, "Modul2/AI sicherer Bereich"=w63, "Modul3/AI sicherer Bereich"=w62, "Traps/Machs sicherer Bereich"=w61, w55, "Metavariablen grüner Bereich"=w54) -> (w60:T18)  [unwired: 1 in]
      n17 = Concatenate Strings("?SE0,SETP,2200" ("string"), "\r\n") -> (w71:string)
      n18 = Concatenate Strings("?SE0,SETP,2300" ("string"), "\r\n") -> (w78:string)
      n19 = String To Byte Array(string=w78) -> (unsigned byte array=w83:u8[])
      n20 = Join Numbers(hi=w83, lo=u8 6) -> ((hi.lo)=w81:u16[])
      n21 = String To Byte Array(string=w71) -> (unsigned byte array=w73:u8[])
      n22 = Join Numbers(hi=w73, lo=u8 5) -> ((hi.lo)=w70:u16[])
      n23 = xnode "Invoke Method"("FPGA VI Reference In"=w68, "Data"=w70) -> ("FPGA VI Reference Out"=w76:refnum<k20>)  [unwired: 2 in, 2 out]
      n24 = xnode "Invoke Method"("FPGA VI Reference In"=w76, "Data"=w81) -> ("FPGA VI Reference Out"=w67:refnum<k20>)  [unwired: 2 in, 2 out]
      n25 = global write "GVProbenvol.vi" "Probenvol.1"(w139) -> ()
      n26 = global write "GVProbenvol.vi" "Probenvol.2"(w139) -> ()
      n27 = global write "GVECDs.vi" "ECD1MW"(w146) -> ()
      n28 = global write "GVECDs.vi" "ECD2MW"(w146) -> ()
      n29 = global write "GVECDs.vi" "ECD1Empfangen?"(w147) -> ()
      n30 = global write "GVECDs.vi" "ECD2Empfangen?"(w147) -> ()
      n31 = property on="dargestellte Größe 2" class="Ring (strict)"("AllowUndefVals"=w241) -> ()  [unwired: 2 in, 2 out]
      n32 = property on="Zeitachse2" class="Ring (strict)"("AllowUndefVals"=w241) -> ()  [unwired: 2 in, 2 out]
      n33 = property on="Zeitachse1" class="Ring (strict)"("AllowUndefVals"=w241) -> ()  [unwired: 2 in, 2 out]
      n34 = property on="dargestellte Größe 1" class="Ring (strict)"("AllowUndefVals"=w241) -> ()  [unwired: 2 in, 2 out]
      n35 = property on="Methode" class="Ring (strict)"("AllowUndefVals"=w241) -> ()  [unwired: 2 in, 2 out]
      n36 = local write "global stop RT"(w242) -> ()
      n37 = global write "gvbooleschRT.vi" "global stop RT"(w242) -> ()
      n38 = global write "GVZeitenZyklen.vi" "ZyklusNummern"(w140) -> ()
      n39 = global write "GVZeitenZyklen.vi" "ZyklusNummernGesamt"(w140) -> ()
      n40 = global write "GVZeitenZyklen.vi" "Big Ben, Methodenzeit, Zykluszeit0, Zykluszeit1, Zykluszeit2A, Zykluszeit2B"(w143) -> ()
      n41 = property on="Methode" class="Ring (strict)"("Value"=w122) -> ()  [unwired: 2 in, 2 out]
      n42 = call "MPVSenden-01-17.vi"("Ventilposition"=0, "FPGA VI Reference In"=w67) -> ("FPGA VI Reference Out"=w65:refnum<k20>)  [unwired: 1 in, 2 out]
      n43 = Initialize Array(-1.0 ("Element"), 6 ("Dimension")) -> (w149:dbl[])
      n44 = Initialize Array(FALSE, 10 ("Dimension")) -> (w156:bool[])
      n45 = Initialize Array(-1.0 ("Element"), 96 ("Dimension")) -> (w150:dbl[])
      n46 = global write "GVZwangs.vi" "ZwangsFPGABoolesch!"(w156) -> ()
      n47 = global write "GVZwangs.vi" "ZwangsFPGABoolesch?"(w156) -> ()
      n48 = global write "GVTrapsMachs.vi" "Traps/Machs"(w149) -> ()
      n49 = global write "GVAIs.vi" "AIs"(w150) -> ()
      n50 = for {
        tunnel: w155 -> [w394] mode=indexing
        tunnel: [w391] -> w154 mode=indexing
        tunnel: [w389] -> w153 mode=indexing
        n51 = Initialize Array(0.0 ("Element"), w394) -> (w392:dbl[])
        n52 = Initialize Array(FALSE, w394) -> (w390:bool[])
        n53 = Bundle(w392) -> (w391:cluster{dbl[]})  [unwired: 1 in]
        n54 = Bundle(w390) -> (w389:cluster{bool[]})  [unwired: 1 in]
      }
      n55 = Bundle("DIOsMod0Name"=w96, "DIOsMod1Name"=w97, "DIOsMod2AName"=w95, "DIOsMod2BName"=w94, "ReglerNameMod0"=w113, "ReglerNameMod1"=w112, "ReglerNameMod2A"=w111, "ReglerNameMod2B"=w110, "LangsameHeizungen"=w182) -> (w244:T19)  [unwired: 1 in]
      n56 = Build Array (concatenate)(w113, w112, w111, w110) -> (w137:string[])
      n57 = Build Array (concatenate)(w204, w203, w202, w201) -> (w255:string[])
      n58 = Build Array (concatenate)(w208, w207, w206, w205) -> (w256:string[])
      n59 = Build Array (concatenate)(w200, w199, w198, w197) -> (w248:dbl[])
      n60 = Build Array (concatenate)(w196, w195, w194, w193) -> (w254:string[])
      n61 = Build Array (concatenate)(w113, w112, w111, w110) -> (→"HorstRegler":string[])
      n62 = Array Size(array=w117) -> (size(s)=w116:i32)
      n63 = Build Array(w165, w164, w163, w162) -> (w161:i32[][])
      n64 = Array Size(array=w182) -> (size(s)=w181:i32)
      n65 = Add Array Elements(numeric array=w155) -> (sum=w240:i32)
      n66 = Array Size(array=w152) -> (size(s)=w50:i32)
      n67 = Index Array(array=w123, index=w122) -> (element=w121:T20)
      n68 = Add Array Elements(numeric array=w155) -> (sum=w167:i32)
      n69 = Build Cluster Array(w165, w164, w163, w162) -> (w247:cluster{"DIOsMod2BNr":i32[]}[])
      n70 = Decrement(x=w177) -> (x-1=w176:i32[])
      n71 = Build Array (concatenate)(w188, w187, w186) -> (w128:string[])
      n72 = Index Array(array=w189, index (col)=0 ("Deaktivierter Index (Spalte)")) -> (element=w234:dbl[])  [unwired: 1 in]
      n73 = Index Array(array=w189, index (col)=1 ("Deaktivierter Index (Spalte)")) -> (element=w235:dbl[])  [unwired: 1 in]
      n74 = Index Array(array=w189, index (col)=2 ("Deaktivierter Index (Spalte)")) -> (element=w236:dbl[])  [unwired: 1 in]
      n75 = Initialize Array(FALSE, 6 ("Dimension")) -> (w45:bool[])
      n76 = global write "GVZwangs.vi" "ZwangsSchnelleHeizungen?"(w45) -> ()
      n77 = Initialize Array(0.0, 6 ("Dimension")) -> (w43:dbl[])
      n78 = for {
        tunnel: w247 -> [w419] mode=indexing
        tunnel: [w420] -> w246 mode=indexing
        n79 = Unbundle(w419) -> ("DIOsMod2BNr"=w418:i32[])
        n80 = Array Size(array=w418) -> (size(s)=w420:i32)
      }
      n81 = property on="Methode" class="Ring (strict)"("Strings []"=w249) -> ()  [unwired: 2 in, 2 out]
      n82 = Build Array (concatenate)(w150, w149) -> (w148:dbl[])
      n83 = Array Size(array=w161) -> (size(s)=w160:i32[])
      n84 = Unbundle(w121) -> ("SPMPV"=w120:i32[])  [unwired: 44 out]
      n85 = Open/Create/Replace File(file path (use dialog)=path "c:/fromcriordy.txt" ("Dateipfad (Dialog verwenden)"), operation (0:open)=T14."replace or create" ("Operation (0:Öffnen)")) -> (refnum out=w213:refnum<file>, error out=w214:errorcluster)  [unwired: 4 in, 1 out]
      n86 = Initialize Array(0.0 ("Element"), w167) -> (w166:dbl[])
      n87 = Initialize Array(0.0 ("element"), w116) -> (w114:dbl[])
      n88 = Get Date/Time In Seconds() -> (seconds since 1Jan1904=w108:timestamp)
      n89 = Initialize Array(FALSE, w50) -> (w51:bool[])
      n90 = Multiply(x=w176, y=32) -> (x*y=w179:i32[])
      n91 = Initialize Array(-1.0, w167) -> (w169:dbl[])
      n92 = global write "GVZwangs.vi" "ZwangsSchnelleHeizungen!"(w43) -> ()
      n93 = Array Subset(array=w128, index=32 ("Index"), length=32 ("Länge")) -> (→"AIs2":string[])
      n94 = Array Subset(array=w128, index=0 ("Index"), length=32 ("Länge")) -> (→"AIs1":string[])
      n95 = Array Subset(array=w128, index=64 ("Index"), length=32 ("Länge")) -> (→"AIs3":string[])
      n96 = global write "GVZwangs.vi" "ZwangsLangsameHeizungenAn!"(w51) -> ()
      n97 = global write "GVZwangs.vi" "ZwangsLangsameHeizungenAn?"(w51) -> ()
      n98 = Initialize Array(0.0 ("element"), w50) -> (w48:dbl[])
      n99 = global write "GVHK1Hz.vi" "Mod1Mod2Mod3/AITrapsMachs1Hz"(w148) -> ()
      n100 = global write "GVHorstSP.vi" "HorstSP"(w166) -> ()
      n101 = for {
        tunnel: w160 -> [w399] mode=indexing
        tunnel: [w396] -> w159 mode=indexing
        n102 = Initialize Array(FALSE, w399) -> (w397:bool[])
        n103 = Bundle(w397) -> (w396:cluster{bool[]})  [unwired: 1 in]
      }
      n104 = global write "GVMetavariablen.vi" "Metavariablen"(w114) -> ()
      n105 = global write "GVHeizenLH.vi" "Heizen?LH"(w51) -> ()
      n106 = Add(x=w179, y=w152) -> (x+y=w178:i32[])
      n107 = global write "GVZwangs.vi" "ZwangsLangsameHeizungenSP?"(w51) -> ()
      n108 = Close File(refnum=w213, error in=w214) -> (path=w245:path)  [unwired: 1 out]
      n109 = Format Date/Time String(time format string (%c)="%Y-%m-%d--%H-%M" ("Zeitformatierungs-String (%c)"), seconds (now)=w108) -> (date/time string=w86:string)  [unwired: 1 in]
      n110 = Index Array(array=w120, index=0) -> (element=w118:i32)
      n111 = global write "GVZwangs.vi" "ZwangsLangsameHeizungenSP!"(w48) -> ()
      n112 = global write "GVMWHorst.vi" "MWHorst"(w169) -> ()
      n113 = global write "GVVentilposition.vi" "Ventilposition"(w118) -> ()
      n114 = Build Array (concatenate)(string[] ["Jahr", "Monat", "Tag", "Stunde", "Minute", "Sekunde"] ("Array"), string[] ["Datei Nr.", "Methode Nr.", "Zyklusnr. Mod0", "Zyklusnr. Mod1", "Zyklusnr. Mod2A", "Zyklusnr. Mod2B"], w251, w128, w138, w137, "Probenvolumen1", "Probenvolumen2", "Ventilposition" ("element"), string[] ["CPU Total", "CPU Time critical", "CPU Timed Structures", "CPU High", "CPU Above normal", "CPU Normal", "CPU Background", "CPU Idle", "CPU ISR", "Memory", "SekundenTotalBrutal"]) -> (w253:string[])
      n115 = Build Array (concatenate)(w138, w137) -> (w136:string[])
      n116 = Build Array (concatenate)(w128, w138, w137) -> (w135:string[])
      n117 = Split 1D Array(array=w251, index=2 ("Index")) -> (second subarray=w243:string[])  [unwired: 1 out]
      n118 = Concatenate Strings("HK " ("String"), w86) -> (w90:string)
      n119 = Concatenate Strings("ECD1 " ("String"), w86) -> (w88:string)
      n120 = Concatenate Strings("ECD2 " ("String"), w86) -> (w85:string)
      n121 = property on="dargestellte Größe 1" class="Ring (strict)"("Strings []"=w135) -> ()  [unwired: 2 in, 2 out]
      n122 = property on="Zeitachse2" class="Ring (strict)"("Strings []"=w243) -> ()  [unwired: 2 in, 2 out]
      n123 = property on="Zeitachse1" class="Ring (strict)"("Strings []"=w243) -> ()  [unwired: 2 in, 2 out]
      n124 = property on="dargestellte Größe 3" class="Ring (strict)"("Strings []"=w136) -> ()  [unwired: 2 in, 2 out]
      n125 = global write "GVZwangs.vi" "ZwangsHorst!"(w154) -> ()
      n126 = property on="dargestellte Größe 2" class="Ring (strict)"("Strings []"=w135) -> ()  [unwired: 2 in, 2 out]
      n127 = global write "GVZwangs.vi" "ZwangsHorst?"(w153) -> ()
      n128 = Build Path(base path=w93, name or relative path=w90) -> (appended path=w101:path)
      n129 = Build Path(base path=w107, name or relative path=w88) -> (appended path=w103:path)
      n130 = Build Path(base path=w106, name or relative path=w85) -> (appended path=w105:path)
      n131 = Create Folder(path (use dialog)=w101) -> (created path=w100:path)  [unwired: 2 in, 2 out]
      n132 = Create Folder(path (use dialog)=w103) -> (created path=w102:path)  [unwired: 2 in, 2 out]
      n133 = Create Folder(path (use dialog)=w105) -> (created path=w104:path)  [unwired: 2 in, 2 out]
      n134 = global write "GVZwangs.vi" "ZwangsDIO!"(w159) -> ()
      n135 = global write "GVZwangs.vi" "ZwangsDIO?"(w159) -> ()
      n136 = case shown="True" w124 {
        tunnel: [w410 w415] -> w227
        tunnel: [w410 w414] -> w226
        tunnel: w100 -> [_ w413]
        tunnel: w185 -> [_ w412]
        tunnel: w122 -> [_ w411]
        frame False {
          w410 = refnum<k34> refnum ("tdms1")
        }
        frame True {
          n137 = call "TDMS0.vi"("Startmethode"=w411, "Dateiname"=w412, "Dateiordner"=w413) -> ("tdms1"=w414:refnum<k34>, "tdms0"=w415:refnum<k34>)
          n138 = global write "GVaktuelleTDMS.vi" "aktuelleTDMS-DateiHK"(w415) -> ()
        }
      }
      n139 = case shown="True" w124 {
        tunnel: [w400 w409] -> w225
        tunnel: [w400 w408] -> w224
        tunnel: [w400 w407] -> w223
        tunnel: [w400 w406] -> w222
        tunnel: w102 -> [_ w405]
        tunnel: w184 -> [_ w404]
        tunnel: w104 -> [_ w403]
        tunnel: w183 -> [_ w402]
        tunnel: w122 -> [_ w401]
        frame False {
          w400 = refnum<k34> refnum ("tdms0")
        }
        frame True {
          n140 = call "TDMS0.vi"("Startmethode"=w401, "Dateiname"=w404, "Dateiordner"=w405) -> ("tdms1"=w408:refnum<k34>, "tdms0"=w409:refnum<k34>)
          n141 = call "TDMS0.vi"("Startmethode"=w401, "Dateiname"=w402, "Dateiordner"=w403) -> ("tdms1"=w406:refnum<k34>, "tdms0"=w407:refnum<k34>)
          n142 = global write "GVaktuelleTDMS.vi" "aktuelleTDMS-DateiECD1"(w409) -> ()
          n143 = global write "GVaktuelleTDMS.vi" "aktuelleTDMS-DateiECD2"(w407) -> ()
        }
      }
      n144 = Open/Create/Replace File(file path (use dialog)=path "c:/fromcriocmd.txt" ("Pfad MS-Datei CRIO"), operation (0:open)=T14."replace or create" ("Operation (0:Öffnen)")) -> (refnum out=w219:refnum<file>, error out=w218:errorcluster)  [unwired: 4 in, 1 out]
      n145 = call "AIKoeffSortieren.vi"("Modul3/AI koeff"=w190, "Modul2/AI koeff"=w191, "Modul1/AI koeff"=w192) -> ("P0"=w231:dbl[], "P1"=w232:dbl[], "P2"=w233:dbl[])
      n146 = Write to Text File(file (use dialog)=w219, text="time=yyyymmddhhmmss\ncycle=005\ninfo=1234567890123456789012345678901234567890123456789012345678901234567890123456789012345678901234567890\nlength=100\ncmd=cycle" ("Text0 MS-Datei"), error in=w218) -> (refnum out=w216:refnum<file>, error out=w215:errorcluster)  [unwired: 1 in, 1 out]
      n147 = Bundle("created path"=w100, "created path"=w102, "created path"=w104, "Dateiname Housekeeping"=w185, "DateinameECD1"=w184, "DateinameECD2"=w183, "tdms0"=w227, "tdms1"=w226, "tdms0"=w225, "tdms1"=w224, "tdms0"=w223, "tdms1"=w222) -> (w228:T21)  [unwired: 1 in]
      n148 = Close File(refnum=w216, error in=w215) -> (path=w210:path)  [unwired: 1 out]
      n149 = property on="Handbetrieb" class="Bool (strict)"("Value"=FALSE ("Handbetrieb")) -> ()  [unwired: 2 in, 2 out]
      "schnelle Heizungen" <- string[] ["Trap1 [°C]", "Trap2 [°C]", "PreCol1 [°C]", "PreCol2 [°C]", "MainCol1 [°C]", "MainCol2 [°C]"]
    }
    frame #1 {
      w429 = dbl[] [-1.0]
      w500 = 0
      w475 = 0 ("Zyklusnummer1")
      n150 = while {
        tunnel: w453 -> [w882]
        tunnel: w522 -> [w881]
        tunnel: w521 -> [w880]
        tunnel: w520 -> [w879]
        shift-right: [w878] -> _
        shift-left: errorcluster {"status"=FALSE, "code"=0, "source"=""} ("error out") -> [w877]
        stop <- w883 stop-if-true
        n151 = call "AIsFIFORT-01-17.vi"("FPGA VI Reference In"=w882, "P2"=w881, "P1"=w880, "P0"=w879, "error in"=w877) -> ("error out"=w878:errorcluster)
        "AIsFIFOread" <- w878
        n152 = global read "gvbooleschRT.vi" "global stop RT"() -> (w883:bool)
      }
      n153 = Add Array Elements(numeric array=w449) -> (sum=w448:i32)
      n154 = Array Size(array=w457) -> (size(s)=w478:i32)
      n155 = Unbundle(w474) -> ("created path"=w473:path, "created path"=w471:path, "created path"=w470:path, "Dateiname Housekeeping"=w472:string, "DateinameECD1"=w469:string, "DateinameECD2"=w468:string, "tdms0"=w467:refnum<k34>, "tdms1"=w466:refnum<k34>, "tdms0"=w465:refnum<k34>, "tdms1"=w464:refnum<k34>, "tdms0"=w463:refnum<k34>, "tdms1"=w462:refnum<k34>)
      n156 = while {
        stop <- w1332 stop-if-true
        w1326 = 10.0
        n157 = call "Warten2"("Count(mSec)"=u32 1000) -> ()  [unwired: 1 out]
        n158 = global read "gvbooleschRT.vi" "global stop RT"() -> (w1332:bool)
        n159 = global read "GVTrapsMachs.vi" "Traps/Machs"() -> (w1322:dbl[])
        n160 = global read "GVAIs.vi" "AIs"() -> (w1323:dbl[])
        n161 = for {
          N: 9 -> [_]
          shift-right: [w1335] -> w1329
          shift-left: w1323 -> [w1336]
          shift-right: [w1333] -> w1327
          shift-left: w1322 -> [w1334]
          n162 = flat-sequence {
            tunnel: w1336 -> [w1343]
            tunnel: [w1342] -> w1335
            tunnel: w1334 -> [w1341]
            tunnel: [w1340] -> w1333
            frame #0 {
              n163 = call "Warten28"("Count(mSec)"=u32 100) -> ()  [unwired: 1 out]
            }
            frame #1 {
              n164 = global read "GVAIs.vi" "AIs"() -> (w1339:dbl[])
              n165 = Add(x=w1343, y=w1339) -> (x+y=w1342:dbl[])
              n166 = global read "GVTrapsMachs.vi" "Traps/Machs"() -> (w1338:dbl[])
              n167 = Add(x=w1338, y=w1341) -> (x+y=w1340:dbl[])
            }
          }
        }
        n168 = Divide(x=w1329, y=w1326) -> (x/y=w1328:dbl[])
        n169 = Divide(x=w1327, y=w1326) -> (x/y=w1325:dbl[])
        n170 = Build Array (concatenate)(w1328, w1325) -> (w1324:dbl[])
        n171 = global write "GVHK1Hz.vi" "Mod1Mod2Mod3/AITrapsMachs1Hz"(w1324) -> ()
      }
      n172 = while {
        shift-right: ["Methode"] -> _
        shift-left: w526 -> [w1346]
        stop <- w1348 stop-if-true
        n173 = call "Bis zum nächsten Vielfachen warten7"("Count(mSec)"=u32 1000) -> ()  [unwired: 1 out]
        n174 = Not Equal?(x=w1346, y="Methode") -> (x != y?=w1344:bool)
        n175 = global write "GVMethodenwechsel.vi" "Methodenwechsel?"(w1344) -> ()
        n176 = global read "gvbooleschRT.vi" "global stop RT"() -> (w1348:bool)
      }
      n177 = Index Array(array=w450, index #1=0 ("Index"), index #2=1 ("Index"), index #3=2 ("Index"), index #4=3 ("Index")) -> (element #1=w489:i32, element #2=w488:i32, element #3=w491:i32, element #4=w490:i32)
      n178 = while {
        tunnel: w453 -> [w884]
        tunnel: w428 -> [w889]
        tunnel: w427 -> [w888]
        tunnel: w426 -> [w887]
        shift-right: [w886] -> _
        shift-left: errorcluster {"status"=FALSE, "code"=0, "source"=""} ("error out") -> [w885]
        stop <- w891 stop-if-true
        n179 = call "TrapsMachMitteln-01-17.vi"("FPGA VI Reference In"=w884, "Traps/MachKoeff2"=w889, "Traps/MachKoeff1"=w888, "Traps/MachKoeff0"=w887, "error in"=w885) -> ("error out"=w886:errorcluster)
        "MWTrapsMachs" <- w886
        n180 = global read "gvbooleschRT.vi" "global stop RT"() -> (w891:bool)
        n181 = call "Bis zum nächsten Vielfachen warten16"("Count(mSec)"=u32 100) -> ()  [unwired: 1 out]
      }
      n182 = call <vilib>:"Space Constant.vi"() -> ("String"=w435:string)
      n183 = case shown="True" TRUE ("ECDSpeichern") {
        frame False {
        }
        frame True {
          w817 = dbl[] []
          n184 = global read "GVaktuelleTDMS.vi" "aktuelleTDMS-DateiECD1"() -> (w818:refnum<k34>)
          n185 = while {
            shift-right: [w830] -> _
            shift-left: w817 -> [w834]
            shift-right: [w823] -> _
            shift-left: w817 -> [w827]
            shift-right: [w829] -> _
            shift-left: w818 -> [w832]
            tunnel: w817 -> [w826]
            shift-right: [w820] -> _
            shift-left: errorcluster {"status"=FALSE, "code"=0, "source"=""} ("error IO") -> [w819]
            stop <- w839 stop-if-true
            n186 = global read "GVaktuelleTDMS.vi" "aktuelleTDMS-DateiECD1"() -> (w829:refnum<k34>)
            n187 = global read "GVaktuelleTDMS.vi" "aktuelleTDMS-DateiECD2"() -> (w837:refnum<k34>)
            n188 = call "Bis zum nächsten Vielfachen warten3"("Count(mSec)"=u32 500) -> ()  [unwired: 1 out]
            n189 = global read "GVECDs.vi" "ECD1MW"() -> (w833:dbl[])
            n190 = global read "GVECDs.vi" "ECD2MW"() -> (w824:dbl[])
            n191 = Equal?(x=w832, y=w829) -> (x = y?=w825:bool)
            n192 = Build Array (concatenate)(w834, w833) -> (w831:dbl[])
            n193 = Build Array (concatenate)(w827, w824) -> (w828:dbl[])
            n194 = TDMS Write(0:w829, 7:"ECD1", 9:w833, 11:w819) -> (15:w822:errorcluster)  [unwired: 2 in, 3 out]
            n195 = TDMS Write(0:w837, 7:"ECD2", 9:w824, 11:w819) -> (15:w821:errorcluster)  [unwired: 2 in, 3 out]
            n196 = Select(t=w828, s=w825, f=w826) -> (s? t:f=w823:dbl[])
            n197 = Select(t=w831, s=w825, f=w826) -> (s? t:f=w830:dbl[])
            n198 = Merge Errors(w822, w821) -> (w820:errorcluster)
            "TDMSwriteECD" <- w820
            n199 = global write "GVChroms.vi" "ECD2Chrom"(w823) -> ()
            n200 = global write "GVChroms.vi" "ECD1Chrom"(w830) -> ()
            n201 = global read "gvbooleschRT.vi" "global stop RT"() -> (w839:bool)
          }
        }
      }
      n202 = while {
        shift-right: [w533] -> _
        shift-left: w429 -> [w535]
        shift-right: [w532] -> _
        shift-left: w429 -> [w534]
        stop <- w537 stop-if-true
        n203 = call "Bis zum nächsten Vielfachen warten"("Count(mSec)"=u32 100) -> ()  [unwired: 1 out]
        n204 = case shown="True" "An/Aus" {
          tunnel: w535 -> [w539 w555]
          tunnel: w534 -> [w538 w554]
          tunnel: [w539 w548] -> w533
          tunnel: [w538 w547] -> w532
          frame False {
          }
          frame True {
            w551 = dbl[] [] ("t")
            n205 = global read "GVMWHorst.vi" "MWHorst"() -> (w544:dbl[])
            n206 = global read "GVTrapsMachs.vi" "Traps/Machs"() -> (w545:dbl[])
            n207 = Build Array (concatenate)(w545, w544) -> (w543:dbl[])
            n208 = Index Array(array=w543, index="dargestellte Größe 3") -> (element=w556:dbl)
            n209 = Build Array (concatenate)(w555, w556) -> (w549:dbl[])
            n210 = Select(t=w551, s="TafelWischen!", f=w549) -> (s? t:f=w548:dbl[])
            n211 = global read "GVZeitenZyklen.vi" "Big Ben, Methodenzeit, Zykluszeit0, Zykluszeit1, Zykluszeit2A, Zykluszeit2B"() -> (w542:dbl[])
            n212 = Index Array(array=w542, index=1 ("Index")) -> (element=w540:dbl)
            n213 = Build Array (concatenate)(w554, w540) -> (w550:dbl[])
            n214 = Select(t=w551, s="TafelWischen!", f=w550) -> (s? t:f=w547:dbl[])
            n215 = Bundle(w550, w549) -> (→"schnelleAnzeige":cluster{dbl[], dbl[]})  [unwired: 1 in]
          }
        }
        n216 = global read "gvbooleschRT.vi" "global stop RT"() -> (w537:bool)
      }
      n217 = case shown="True" TRUE ("HKSpeichern") {
        tunnel: w524 -> [_ w870]
        frame False {
        }
        frame True {
          n218 = while {
            tunnel: w870 -> [w874]
            shift-right: [w872] -> _
            shift-left: errorcluster {"status"=FALSE, "code"=0, "source"=""} ("error out") -> [w871]
            stop <- w876 stop-if-true
            n219 = local read "Methode"() -> (w873:i32)
            n220 = call "Bis zum nächsten Vielfachen warten2"("Count(mSec)"=u32 1000) -> ()  [unwired: 1 out]
            n221 = call "HKinTDMS-01-16.vi"("Methode"=w873, "error in (no error)"=w871, "Kanäle"=w874) -> ("error out"=w872:errorcluster)
            "TDMSwriteHK" <- w872
            n222 = global read "gvbooleschRT.vi" "global stop RT"() -> (w876:bool)
          }
        }
      }
      n223 = for {
        N: 1 -> [_]
        tunnel: w453 -> [w892]
        tunnel: [w892] -> w480
        n224 = call "Warten8"("Count(mSec)"=u32 100) -> ()  [unwired: 1 out]
      }
      n225 = global read "GVVentilposition.vi" "Ventilposition"() -> (w459:i32)
      n226 = Build Array(w435) -> (w434:string[])
      n227 = Initialize Array(-1 ("Element"), 4 ("Dimension")) -> (w451:i32[])
      n228 = case shown="True" TRUE {
        tunnel: w475 -> [_ w849]
        tunnel: w473 -> [_ w848]
        tunnel: w472 -> [_ w847]
        tunnel: w467 -> [_ w846]
        tunnel: w466 -> [_ w845]
        frame False {
        }
        frame True {
          w840 = errorcluster {"status"=FALSE, "code"=0, "source"=""} ("error out TDMSopen")
          n229 = while {
            shift-right: [w854] -> w844
            shift-left: w846 -> [w856]
            shift-right: [w865] -> w843
            shift-left: w845 -> [w858]
            shift-right: [w860] -> _
            shift-left: w849 -> [w866]
            tunnel: w847 -> [w862]
            tunnel: w848 -> [w863]
            shift-right: [w853] -> w842
            shift-left: w840 -> [w851]
            shift-right: [w852] -> w841
            shift-left: w840 -> [w850]
            stop <- w868 stop-if-true
            n230 = global read "GVZeitenZyklen.vi" "ZyklusNummernGesamt"() -> (w855:i32[])
            n231 = call "Bis zum nächsten Vielfachen warten5"("Count(mSec)"=u32 500) -> ()  [unwired: 1 out]
            n232 = Index Array(array=w855, index=1 ("Index")) -> (element=w860:i32)
            n233 = Greater?(x=w860, y=w866) -> (0:w859:bool)
            n234 = Select(t=w858, s=w859, f=w856) -> (s? t:f=w857:refnum<k34>)
            n235 = local read "Methode"() -> (w864:i32)
            n236 = global write "GVaktuelleTDMS.vi" "aktuelleTDMS-DateiHK"(w857) -> ()
            n237 = call "AktuelleTDMS.vi"("AktuelleTDMS"=w856, "error in TDMSopen"=w851, "Dateiordner"=w863, "NächsteTDMS"=w858, "NeuerZyklus?"=w859, "Methodennummer"=w864, "Zyklnumges"=w860, "error in TDMSclose"=w850, "Dateiname"=w862) -> ("AktuelleTDMS"=w854:refnum<k34>, "error out TDMSopen"=w853:errorcluster, "error out TDMSclose"=w852:errorcluster, "NächsteTDMS"=w865:refnum<k34>)  [unwired: 3 in]
            "TDMSopenHK" <- w853
            "TDMScloseHK" <- w852
            n238 = global read "gvbooleschRT.vi" "global stop RT"() -> (w868:bool)
          }
          n239 = TDMS Close(8:w842, 11:w844) -> ()  [unwired: 2 out]
          n240 = TDMS Close(8:w841, 11:w843) -> ()  [unwired: 2 out]
        }
      }
      n241 = case shown="True" TRUE {
        tunnel: w475 -> [_ w777]
        tunnel: w471 -> [_ w776]
        tunnel: w470 -> [_ w775]
        tunnel: w469 -> [_ w774]
        tunnel: w468 -> [_ w773]
        tunnel: w465 -> [_ w772]
        tunnel: w464 -> [_ w771]
        tunnel: w463 -> [_ w770]
        tunnel: w462 -> [_ w769]
        frame False {
        }
        frame True {
          w762 = errorcluster {"status"=FALSE, "code"=0, "source"=""} ("error out TDMSopen")
          n242 = while {
            shift-right: [w801] -> w768
            shift-left: w772 -> [w803]
            shift-right: [w811] -> w767
            shift-left: w771 -> [w805]
            shift-right: [w809] -> _
            shift-left: w777 -> [w812]
            tunnel: w776 -> [w808]
            tunnel: w774 -> [w807]
            shift-right: [w800] -> w763
            shift-left: w762 -> [w798]
            shift-right: [w799] -> w764
            shift-left: w762 -> [w797]
            stop <- w814 stop-if-true
            n243 = global read "GVZeitenZyklen.vi" "ZyklusNummernGesamt"() -> (w802:i32[])
            n244 = call "Bis zum nächsten Vielfachen warten4"("Count(mSec)"=u32 500) -> ()  [unwired: 1 out]
            n245 = Index Array(array=w802, index=2 ("Index")) -> (element=w809:i32)
            n246 = Greater?(x=w809, y=w812) -> (0:w806:bool)
            n247 = Select(t=w805, s=w806, f=w803) -> (s? t:f=w804:refnum<k34>)
            n248 = local read "Methode"() -> (w810:i32)
            n249 = global write "GVaktuelleTDMS.vi" "aktuelleTDMS-DateiECD1"(w804) -> ()
            n250 = call "AktuelleTDMS.vi"("AktuelleTDMS"=w803, "error in TDMSopen"=w798, "Dateiordner"=w808, "NächsteTDMS"=w805, "NeuerZyklus?"=w806, "Methodennummer"=w810, "Zyklnumges"=w809, "error in TDMSclose"=w797, "Dateiname"=w807) -> ("AktuelleTDMS"=w801:refnum<k34>, "error out TDMSopen"=w800:errorcluster, "error out TDMSclose"=w799:errorcluster, "NächsteTDMS"=w811:refnum<k34>)  [unwired: 3 in]
            "TDMSopenECD1" <- w800
            "TDMScloseECD1" <- w799
            n251 = global read "gvbooleschRT.vi" "global stop RT"() -> (w814:bool)
          }
          n252 = while {
            shift-right: [w791] -> w766
            shift-left: w770 -> [w783]
            shift-right: [w792] -> w765
            shift-left: w769 -> [w785]
            shift-right: [w789] -> _
            shift-left: w777 -> [w793]
            tunnel: w775 -> [w788]
            tunnel: w773 -> [w787]
            shift-right: [w781] -> _
            shift-left: w762 -> [w779]
            shift-right: [w780] -> _
            shift-left: w762 -> [w778]
            stop <- w795 stop-if-true
            n253 = global read "GVZeitenZyklen.vi" "ZyklusNummernGesamt"() -> (w782:i32[])
            n254 = call "Bis zum nächsten Vielfachen warten6"("Count(mSec)"=u32 500) -> ()  [unwired: 1 out]
            n255 = Index Array(array=w782, index=3 ("Index")) -> (element=w789:i32)
            n256 = Greater?(x=w789, y=w793) -> (0:w786:bool)
            n257 = Select(t=w785, s=w786, f=w783) -> (s? t:f=w784:refnum<k34>)
            n258 = local read "Methode"() -> (w790:i32)
            n259 = global write "GVaktuelleTDMS.vi" "aktuelleTDMS-DateiECD2"(w784) -> ()
            n260 = call "AktuelleTDMS.vi"("AktuelleTDMS"=w783, "error in TDMSopen"=w779, "Dateiordner"=w788, "NächsteTDMS"=w785, "NeuerZyklus?"=w786, "Methodennummer"=w790, "Zyklnumges"=w789, "error in TDMSclose"=w778, "Dateiname"=w787) -> ("AktuelleTDMS"=w791:refnum<k34>, "error out TDMSopen"=w781:errorcluster, "error out TDMSclose"=w780:errorcluster, "NächsteTDMS"=w792:refnum<k34>)  [unwired: 3 in]
            "TDMSopenECD2" <- w781
            "TDMScloseECD2" <- w780
            n261 = global read "gvbooleschRT.vi" "global stop RT"() -> (w795:bool)
          }
          n262 = TDMS Close(8:w763, 11:w768) -> ()  [unwired: 2 out]
          n263 = TDMS Close(8:w764, 11:w767) -> ()  [unwired: 2 out]
          n264 = TDMS Close(11:w766) -> ()  [unwired: 1 in, 2 out]
          n265 = TDMS Close(11:w765) -> ()  [unwired: 1 in, 2 out]
        }
      }
      n266 = Add(x=w491, y=w490) -> (x+y=w487:i32)
      n267 = Bundle(w434, w434, w434) -> (w498:cluster{string[], string[], string[]})  [unwired: 1 in]
      n268 = Index Array(array=w444, index=w442) -> (element=w443:T20)
      n269 = Initialize Array(cluster{"output high":dbl, "output low":dbl} {"output high"=99999.0, "output low"=0.0} ("output range"), w478) -> (w458:cluster{"output high":dbl, "output low":dbl}[])
      n270 = Concatenate Strings("?SE0,GDATA" ("Schreibpuffer"), "\r") -> (w430:string)
      n271 = Build Array(w489, w488, w487) -> (w486:i32[])
      n272 = while {
        tunnel: w525 -> [w1019]
        shift-right: [w1018] -> _
        shift-left: w444 -> [w1000]
        tunnel: w458 -> [w1017]
        tunnel: w457 -> [w1016]
        tunnel: w453 -> [w1015]
        tunnel: w456 -> [w1014]
        tunnel: w455 -> [w1013]
        shift-right: [w1007] -> _
        shift-left: 0 -> [w1012]
        tunnel: w453 -> [w1011]
        tunnel: w452 -> [w1010]
        shift-right: [w1006] -> _
        shift-left: w451 -> [w1009]
        tunnel: w450 -> [w1001]
        tunnel: w449 -> [w1002]
        tunnel: w448 -> [w1003]
        tunnel: w447 -> [w1004]
        tunnel: w446 -> [w1005]
        tunnel: w445 -> [w1008]
        shift-right: [w923] -> _
        shift-left: w443 -> [w922]
        tunnel: w428 -> [w901]
        tunnel: w427 -> [w905]
        tunnel: w426 -> [w911]
        tunnel: w421 -> [w894]
        i -> [w926]
        stop <- w1020 stop-if-true
        w912 = 0  # ZeileMainMach2
        w913 = 0  # ZeileMainMach1
        w968 = FALSE
        w967 = 0.0
        w969 = 0  # ZeilennummerMPV
        w973 = cluster{dbl[], dbl[]} {[], []}
        w982 = dbl[] []
        w986 = 0  # ZeilePreMach2
        w987 = 0  # ZeilePreMach1
        w988 = 0  # ZeileFPGAFixp
        w989 = 0  # ZeileFPGAPID
        w990 = 0  # ZeileFPGABoolesch
        w991 = i32[] [0, 0, 0, 0]  # ZeilennummernHorst
        w992 = i32[] [0, 0, 0, 0]  # ZeilennummernDIOs
        n273 = Unbundle(w922) -> ("Zykluslängen [s]"=w966:dbl[], "ZeitpktDIOsMod0"=w965:dbl[], "ZeitpktDIOsMod1"=w964:dbl[], "ZeitpktDIOsMod2A"=w963:dbl[], "ZeitpktDIOsMod2B"=w962:dbl[], "DIOsSPMod0"=w961:bool[][], "DIOsSPMod1"=w960:bool[][], "DIOsSPMod2A"=w959:bool[][], "DIOsSPMod2B"=w958:bool[][], "Mod0HorstZeitpkt"=w957:dbl[], "Mod1HorstZeitpkt"=w956:dbl[], "Mod2AHorstZeitpkt"=w955:dbl[], "Mod2BHorstZeitpkt"=w954:dbl[], "HorstSPMod0"=w953:dbl[][], "HorstSPMod1"=w952:dbl[][], "HorstSPMod2A"=w951:dbl[][], "HorstSPMod2B"=w950:dbl[][], "LHSetpoints"=w949:dbl[], "LHHeizen?"=w948:bool[], "ZPktFPGABoolesch"=w947:dbl[], "FPGABoolesch"=w946:bool[][], "ZeitpktFPGAPID"=w945:dbl[], "FPGAPID"=w944:T22, "ZeitpktFPGAFixp"=w943:dbl[], "SHSetpoints"=w942:dbl[][], "t_PreMach1"=w941:dbl[], "T_PreMach1"=w940:dbl[], "t_PreMach2"=w939:dbl[], "T_PreMach2"=w938:dbl[], "PIDs für \"träge\" Heizungen"=w937:T23, "Zwangsbedingungen"=w936:dbl[][], "Dateien fürs MS schicken?"=w935:bool, "ZeitpunkteMPV"=w934:dbl[], "SPMPV"=w933:i32[], "ZeitpktMS-1"=w932:dbl, "ZeitpktMS-2"=w931:dbl, "Int.Start1"=w930:dbl, "Int.Stop1"=w929:dbl, "Int.Start2"=w928:dbl, "Int.Stop2"=w927:dbl, "t_MainMach1"=w921:dbl[], "T_MainMach1"=w920:dbl[], "t_MainMach2"=w919:dbl[], "T_MainMach2"=w918:dbl[])  [unwired: 1 out]
        n274 = Add(x=w1009, y=1) -> (x+y=w977:i32[])
        n275 = Array Subset(array=w911, index=2 ("Index"), length=4 ("Länge")) -> (w908:dbl[])
        n276 = Array Subset(array=w905, index=2 ("Index"), length=4 ("Länge")) -> (w904:dbl[])
        n277 = Array Subset(array=w901, index=2 ("Index"), length=4 ("Länge")) -> (w900:dbl[])
        n278 = local read "Methode"() -> (w925:i32)
        n279 = while {
          tunnel: w1016 -> [w1072]
          tunnel: w1017 -> [w1074]
          tunnel: w1015 -> [w1069]
          tunnel: w949 -> [w1073]
          tunnel: w937 -> [w1075]
          shift-right: [w1071] -> _
          shift-left: errorcluster {"status"=FALSE, "code"=0, "source"=""} ("error out") -> [w1070]
          stop <- w1076 stop-if-true
          n280 = call "LH-01-17.vi"("FPGA VI Reference In"=w1069, "OutputRange"=w1074, "LHSetpoints"=w1073, "AIsLH"=w1072, "error in"=w1070, "PIDs für \"träge\" Heizungen"=w1075) -> ("error out"=w1071:errorcluster)  [unwired: 1 in]
          "LH" <- w1071
          n281 = call "Bis zum nächsten Vielfachen warten12"("Count(mSec)"=u32 100) -> ()  [unwired: 1 out]
          n282 = local read "veränderte Methode benutzen"() -> (w1077:bool)
          n283 = global read "GVMethodenwechsel.vi" "Methodenwechsel?"() -> (w1078:bool)
          n284 = global read "gvbooleschRT.vi" "global stop RT"() -> (w1079:bool)
          n285 = Compound Arithmetic op=OR(w1079, w1078, w1077) -> (w1076:bool)
        }
        n286 = while {
          tunnel: w1002 -> [w1092]
          tunnel: w1005 -> [w1090]
          tunnel: w1004 -> [w1089]
          tunnel: w1001 -> [w1091]
          tunnel: w1003 -> [w1088]
          tunnel: w936 -> [w1082]
          stop <- w1084 stop-if-true
          n287 = case shown="True" "Handbetrieb" {
            tunnel: w1092 -> [w1101 _]
            tunnel: w1091 -> [w1100 _]
            tunnel: w1090 -> [w1099 _]
            tunnel: w1089 -> [w1098 _]
            tunnel: w1088 -> [w1097 _]
            tunnel: w1082 -> [w1094 _]
            frame False {
              n288 = local read "Methode"() -> (w1096:i32)
              n289 = call "ZwangsbedingungenGV.vi"("AnzahlHorst"=w1099, "AnzahlHorst/Modul"=w1100, "AnzahlLH"=w1098, "AnzahlDIOs/Modul"=w1101, "AnzahlDIOs"=w1097, "Zwangsbedingungen"=w1094, "Methodennummer"=w1096) -> ("Methodennummer"=w1095:i32)  [unwired: 4 in]
              n290 = local write "Methode"(w1095) -> ()
            }
            frame True {
            }
          }
          n291 = call "Bis zum nächsten Vielfachen warten10"("Count(mSec)"=u32 1000) -> ()  [unwired: 1 out]
          n292 = global read "GVMethodenwechsel.vi" "Methodenwechsel?"() -> (w1086:bool)
          n293 = global read "gvbooleschRT.vi" "global stop RT"() -> (w1087:bool)
          n294 = case shown="True" "global stop RT" {
            frame False {
            }
            frame True {
              n295 = global write "gvbooleschRT.vi" "global stop RT"(TRUE ("global stop RT")) -> ()
            }
          }
          n296 = local read "veränderte Methode benutzen"() -> (w1085:bool)
          n297 = Compound Arithmetic op=OR(w1087, w1086, w1085) -> (w1084:bool)
        }
        n298 = Build Cluster Array(w961, w960, w959, w958) -> (w996:cluster{"DIOsSPMod2B":bool[][]}[])
        n299 = Build Cluster Array(w953, w952, w951, w950) -> (w994:cluster{"HorstSPMod2B":dbl[][]}[])
        n300 = Build Cluster Array(w965, w964, w963, w962) -> (w997:cluster{"ZeitpktDIOsMod2B":dbl[]}[])
        n301 = Build Cluster Array(w957, w956, w955, w954) -> (w995:cluster{"Mod2BHorstZeitpkt":dbl[]}[])
        n302 = Bundle(w908, w904, w900) -> (w899:cluster{dbl[], dbl[], dbl[]})  [unwired: 1 in]
        n303 = Equal?(x=w926, y=0) -> (x = y?=w998:bool)
        n304 = global read "GVZeitenZyklen.vi" "ZyklusNummern"() -> (w976:i32[])
        n305 = global read "GVZwangs.vi" "ZwangsHorst?"() -> (w981:cluster{bool[]}[])
        n306 = global read "gvbooleschRT.vi" "global stop RT"() -> (w1020:bool)
        n307 = global read "GVZwangsMPV.vi" "ZwangsMPV?"() -> (w897:bool)
        n308 = global read "GVZwangs.vi" "ZwangsDIO?"() -> (w980:cluster{bool[]}[])
        n309 = global read "GVaktuelleTDMS.vi" "aktuelleTDMS-DateiECD1"() -> (w975:refnum<k34>)
        n310 = global read "GVZwangs.vi" "ZwangsFPGABoolesch?"() -> (w979:bool[])
        n311 = while {
          shift-right: [w1033] -> _
          shift-left: w968 -> [w1037]
          shift-right: [w1032] -> _
          shift-left: w967 -> [w1036]
          shift-right: [w1031] -> _
          shift-left: w968 -> [w1035]
          shift-right: [w1030] -> _
          shift-left: w967 -> [w1034]
          tunnel: w1008 -> [w1029]
          tunnel: w930 -> [w1024]
          tunnel: w929 -> [w1023]
          tunnel: w928 -> [w1022]
          tunnel: w927 -> [w1021]
          stop <- w1026 stop-if-true
          n312 = call "Integrieren.vi"("Integrieren1"=w1037, "Integral1"=w1036, "Integrieren2"=w1035, "Integral2"=w1034, "Int.Start1"=w1024, "Int.Stop1"=w1023, "Int.Start2"=w1022, "HorstProbenflußNr."=w1029, "Int.Stop2"=w1021) -> ("Integrieren1"=w1033:bool, "Integral1"=w1032:dbl, "Integrieren2"=w1031:bool, "Integral2"=w1030:dbl)  [unwired: 7 in]
          n313 = call "Bis zum nächsten Vielfachen warten9"("Count(mSec)"=u32 100) -> ()  [unwired: 1 out]
          n314 = global read "GVMethodenwechsel.vi" "Methodenwechsel?"() -> (w1027:bool)
          n315 = global read "gvbooleschRT.vi" "global stop RT"() -> (w1028:bool)
          n316 = local read "veränderte Methode benutzen"() -> (w1025:bool)
          n317 = Compound Arithmetic op=OR(w1028, w1027, w1025) -> (w1026:bool)
        }
        n318 = while "Zeit" {
          tunnel: w998 -> [w1283]
          tunnel: w966 -> [w1281]
          tunnel: w977 -> [w1276]
          tunnel: [w1275] -> w1006
          shift-right: [w1272] -> _
          shift-left: 0.0 -> [w1273]
          i -> [w1285]
          stop <- w1278 stop-if-true
          n319 = Equal?(x=w1285, y=0) -> (x = y?=w1274:bool)
          n320 = call "Bis zum nächsten Vielfachen warten15"("Count(mSec)"=u32 50) -> ()  [unwired: 1 out]
          n321 = call "BigBen-01-16.vi"("MethodenStartzeit"=w1273, "Methodenstart?"=w1274, "Programmstart?"=w1283, "Zykluslängen [s]"=w1281, "MethodenStartZyklusNummern"=w1276) -> ("MethodenStartzeit"=w1272:dbl, "ZyklusNummernGesamt"=w1275:i32[])  [unwired: 2 in]
          n322 = global read "GVMethodenwechsel.vi" "Methodenwechsel?"() -> (w1277:bool)
          n323 = global read "gvbooleschRT.vi" "global stop RT"() -> (w1282:bool)
          n324 = local read "veränderte Methode benutzen"() -> (w1280:bool)
          n325 = Or(x=w1277, y=w1282) -> (x .or. y?=w1279:bool)
          n326 = Or(x=w1280, y=w1279) -> (x .or. y?=w1278:bool)
        }
        n327 = Bundle(w997, w996, w995, w994, "LHHeizen?"=w948, "ZPktFPGABoolesch"=w947, "FPGABoolesch"=w946, "ZeitpktFPGAPID"=w945, "FPGAPID"=w944, "ZeitpktFPGAFixp"=w943, "SHSetpoints"=w942, "t_PreMach1"=w941, "T_PreMach1"=w940, "t_PreMach2"=w939, "T_PreMach2"=w938, "ZeitpunkteMPV"=w934, "SPMPV"=w933, "t_MainMach1"=w921, "T_MainMach1"=w920, "t_MainMach2"=w919, "T_MainMach2"=w918) -> (w993:T24)  [unwired: 1 in]
        n328 = Index Array(array=w1000, index=w925) -> (element=w924:T20)
        n329 = while {
          tunnel: w1019 -> [w1298]
          shift-right: [w1289] -> _
          shift-left: w924 -> [w1297]
          tunnel: w925 -> [w1295]
          shift-right: [w1287] -> w1018
          shift-left: w1000 -> [w1296]
          tunnel: [w1288] -> w923
          stop <- w1291 stop-if-true
          n330 = call "Bis zum nächsten Vielfachen warten8"("Count(mSec)"=u32 500) -> ()  [unwired: 1 out]
          n331 = global read "GVMethodenwechsel.vi" "Methodenwechsel?"() -> (w1293:bool)
          n332 = global read "gvbooleschRT.vi" "global stop RT"() -> (w1292:bool)
          n333 = case shown="True" "Methode verändern" {
            tunnel: w1298 -> [_ w1320]
            tunnel: w1297 -> [w1317 w1319]
            tunnel: [w1317 w1318] -> w1289
            frame False {
            }
            frame True {
              n334 = call "methodeändern-11-15.vi"("Methode"=w1319, "Namen"=w1320) -> ("Methode"=w1318:T25)  [unwired: 1 in]
              n335 = property on="Methode verändern" class="Bool (strict)"("Value"=FALSE ("Methode verändern")) -> ()  [unwired: 2 in, 2 out]
            }
          }
          n336 = Compound Arithmetic op=OR(w1293, w1292, "veränderte Methode benutzen") -> (w1291:bool)
          n337 = case shown="True" "Methode speichern" {
            tunnel: w1289 -> [_ w1314]
            tunnel: w1296 -> [w1307 w1316]
            tunnel: w1295 -> [_ w1315]
            tunnel: [w1307 w1309] -> w1287
            frame False {
            }
            frame True {
              n338 = Replace Array Subset(array=w1316, new element=w1314, index=w1315) -> (w1309:T13)
              n339 = property on="Methode speichern" class="Bool (strict)"("Value"=FALSE ("Methode speichern")) -> ()  [unwired: 2 in, 2 out]
              n340 = Open/Create/Replace File(file path (use dialog)=path "c:/methoden.perx" ("Dateipfad (Dialog verwenden)"), operation (0:open)=T14."replace" ("Operation (0:Öffnen)")) -> (refnum out=w1311:refnum<file>)  [unwired: 4 in, 2 out]
              n341 = Write to Binary File(file (use dialog)=w1311, data=w1309) -> (refnum out=w1308:refnum<file>)  [unwired: 4 in, 2 out]
              n342 = Close File(refnum=w1308) -> ()  [unwired: 1 in, 2 out]
            }
          }
          n343 = case shown="False" "veränderte Methode benutzen" {
            tunnel: w1289 -> [_ w1304]
            tunnel: [w1301 w1304] -> w1288
            tunnel: w1287 -> [w1303 _]
            frame False {
              n344 = local read "Methode"() -> (w1302:i32)
              n345 = Index Array(array=w1303, index=w1302) -> (element=w1301:T20)
            }
            frame True {
              n346 = flat-sequence {
                frame #0 {
                  n347 = call "Warten"("Count(mSec)"=u32 1100) -> ()  [unwired: 1 out]
                }
                frame #1 {
                  n348 = property on="veränderte Methode benutzen" class="Bool (strict)"("Value"=FALSE ("Methode verändern")) -> ()  [unwired: 2 in, 2 out]
                }
              }
            }
          }
        }
        n349 = Bundle(w982, w982, w982, w982) -> (w983:cluster{dbl[], dbl[], dbl[], dbl[]})  [unwired: 1 in]
        n350 = Bundle("ZyklusNummern"=w976, "ZeilennummernDIOs"=w992, "ZwangsDIO?"=w980, "ZeilennummernHorst"=w991, "ZwangsHorst?"=w981, "ZeileFPGABoolesch"=w990, "ZwangsFPGABoolesch?"=w979, "ZeileFPGAPID"=w989, "ZeileFPGAFixp"=w988, "ZeilePreMach1"=w987, "ZeilePreMach2"=w986, "ZeilennummerMPV"=w969, "ZeileMainMach1"=w913, "ZeileMainMach2"=w912, "ZwangsMPV?"=w897) -> (w985:T26)  [unwired: 1 in]
        n351 = call "arrayDoppelMoppel-11-15.vi"("verdoppeln"=i32[] [0, 1], "Traps/MachsKoeff2"=w901, "Traps/MachsKoeff1"=w905, "Traps/MachsKoeff0"=w911) -> ("Traps/MachsKoeff2"=w914:dbl[], "Traps/MachsKoeff1"=w915:dbl[], "Traps/MachsKoeff0"=w916:dbl[])  [unwired: 5 in]
        n352 = while "ZyklusSteuerung" {
          tunnel: w1010 -> [w1265]
          tunnel: w1011 -> [w1255]
          shift-right: [w1264] -> _
          shift-left: w985 -> [w1258]
          tunnel: w993 -> [w1262]
          tunnel: w916 -> [w1261]
          tunnel: w915 -> [w1260]
          tunnel: w914 -> [w1259]
          tunnel: w899 -> [w1263]
          shift-right: [w1257] -> _
          shift-left: errorcluster {"status"=FALSE, "code"=0, "source"=""} ("error out") -> [w1256]
          stop <- w1267 stop-if-true
          n353 = local read "veränderte Methode benutzen"() -> (w1268:bool)
          n354 = call "Bis zum nächsten Vielfachen warten11"("Count(mSec)"=u32 100) -> ()  [unwired: 1 out]
          n355 = global read "GVMethodenwechsel.vi" "Methodenwechsel?"() -> (w1270:bool)
          n356 = global read "gvbooleschRT.vi" "global stop RT"() -> (w1269:bool)
          n357 = call "ZyklussteuerungGV-01-17.vi"("Traps/MachKoeff0"=w1261, "DIOsNummern"=w1265, "error in"=w1256, "Traps/MachKoeff1"=w1260, "ServosWarmHigh (us)KaltHigh(us)"="ServosWarmHigh (us)KaltHigh(us)", "Traps/MachKoeff2"=w1259, "Schieberegister"=w1258, "Zeitpunkte/Setpoints"=w1262, "FPGA VI Reference In"=w1255, "MachKoeffs"=w1263) -> ("Schieberegister"=w1264:T27, "error out"=w1257:errorcluster)  [unwired: 4 in]
          "Zyklus" <- w1257
          n358 = Compound Arithmetic op=OR(w1270, w1269, w1268) -> (w1267:bool)
        }
        n359 = while {
          shift-right: [w1213] -> _
          shift-left: w983 -> [w1220]
          shift-right: [w1212] -> _
          shift-left: w983 -> [w1219]
          shift-right: [w1210] -> _
          shift-left: T17 {"Zyklus1"=0, "Zeitachse1"=0, "dargestellte Größe 1"=0, "Zyklus2"=0, "Zeitachse2"=0, "dargestellte Größe 2"=0} ("AnzeigeEinstellungen") -> [w1218]
          tunnel: w966 -> [w1188]
          shift-right: [w1184] -> _
          shift-left: w975 -> [w1183]
          shift-right: [w1179] -> _
          shift-left: w973 -> [w1181]
          shift-right: [w1168] -> _
          shift-left: w973 -> [w1180]
          shift-right: ["Detektor"] -> _
          shift-left: 0 ("Detektor") -> [w1177]
          tunnel: w894 -> [w1166]
          stop <- w1224 stop-if-true
          w1189 = 0.0 ("X-Achse.Bereich:Minimum")
          n360 = call "Bis zum nächsten Vielfachen warten14"("Count(mSec)"=u32 1000) -> ()  [unwired: 1 out]
          n361 = global read "GVMWHorst.vi" "MWHorst"() -> (w1117:dbl[])
          "MWHorst" <- w1117
          n362 = case shown="0, Default" "Detektor" {
            tunnel: [w1234 w1246] -> w1179
            tunnel: w1188 -> [w1233 w1248]
            tunnel: "Detektor" -> [w1228 w1242]
            tunnel: [w1232 w1247] -> w1186
            tunnel: [w1231 w1245] -> w1184
            frame 0, Default {
              n363 = Increment(x=w1228) -> (x+1=w1229:i32)
              n364 = Increment(x=w1229) -> (x+1=w1227:i32)
              n365 = global read "GVChroms.vi" "ECD1Chrom"() -> (w1230:dbl[])
              n366 = global read "GVaktuelleTDMS.vi" "aktuelleTDMS-DateiECD1"() -> (w1231:refnum<k34>)
              n367 = Index Array(array=w1233, index=w1227) -> (element=w1232:dbl)
              n368 = Array Size(array=w1230) -> (size(s)=w1236:i32)
              n369 = for {
                N: w1236 -> [_]
                tunnel: [w1237] -> w1235 mode=indexing
                i -> [w1240]
                n370 = To Double Precision Float(number=w1240) -> (double precision float=w1239:dbl)
                n371 = Divide(x=w1239, y=10.0) -> (x/y=w1237:dbl)
              }
              n372 = Bundle(w1235, "ECD1Chrom"=w1230) -> (w1234:cluster{dbl[], "ECD1Chrom":dbl[]})  [unwired: 1 in]
            }
            frame 1 {
              n373 = Increment(x=w1242) -> (x+1=w1243:i32)
              n374 = Increment(x=w1243) -> (x+1=w1241:i32)
              n375 = global read "GVChroms.vi" "ECD2Chrom"() -> (w1244:dbl[])
              n376 = global read "GVaktuelleTDMS.vi" "aktuelleTDMS-DateiECD2"() -> (w1245:refnum<k34>)
              n377 = Index Array(array=w1248, index=w1241) -> (element=w1247:dbl)
              n378 = Array Size(array=w1244) -> (size(s)=w1250:i32)
              n379 = for {
                N: w1250 -> [_]
                tunnel: [w1251] -> w1249 mode=indexing
                i -> [w1254]
                n380 = To Double Precision Float(number=w1254) -> (double precision float=w1253:dbl)
                n381 = Divide(x=w1253, y=10.0) -> (x/y=w1251:dbl)
              }
              n382 = Bundle(w1249, "ECD2Chrom"=w1244) -> (w1246:cluster{dbl[], "ECD2Chrom":dbl[]})  [unwired: 1 in]
            }
          }
          n383 = Equal?(x="Detektor", y=w1177) -> (x = y?=w1176:bool)
          n384 = Subtract(x="HK1YMax", y="HK1YMin") -> (x-y=w1204:dbl)
          n385 = Subtract(x="HK2YMax", y="HK2YMin") -> (x-y=w1199:dbl)
          n386 = Subtract(x="DetYMax", y="DetYMin") -> (x-y=w1194:dbl)
          n387 = Unbundle(w1166) -> ("Modul1/AI sicherer Bereich"=w1159:dbl[][], "Modul2/AI sicherer Bereich"=w1144:dbl[][], "Modul3/AI sicherer Bereich"=w1135:dbl[][], "Traps/Machs sicherer Bereich"=w1126:dbl[][], w1118:dbl[][], "Metavariablen grüner Bereich"=w1109:dbl[][])
          n388 = Index Array(array=w1118, index (col) #1=0 ("disabled index (col)"), index (col) #2=1 ("index (col)")) -> (element #1=w1122:dbl[], element #2=w1121:dbl[])  [unwired: 2 in]
          n389 = Greater Or Equal?(x=w1117, y=w1122) -> (x >= y?=w1120:bool[])
          n390 = Less Or Equal?(x=w1117, y=w1121) -> (x <= y?=w1119:bool[])
          n391 = And(x=w1120, y=w1119) -> (x .and. y?=→"HorstOK?":bool[])
          n392 = global read "GVMethodenwechsel.vi" "Methodenwechsel?"() -> (w1222:bool)
          n393 = global read "GVZeitenZyklen.vi" "ZyklusNummern"() -> (w1191:i32[])
          "ZyklusNummern" <- w1191
          n394 = global read "GVMetavariablen.vi" "Metavariablen"() -> (w1108:dbl[])
          "Metavariablen" <- w1108
          n395 = global read "gvbooleschRT.vi" "global stop RT"() -> (w1223:bool)
          n396 = global read "GVVentilposition.vi" "Ventilposition"() -> (→"Ventilposition":i32)
          n397 = Index Array(array=w1159, index (col) #1=0 ("disabled index (col)"), index (col) #2=1 ("index (col)")) -> (element #1=w1156:dbl[], element #2=w1154:dbl[])  [unwired: 2 in]
          n398 = Index Array(array=w1135, index (col) #1=0 ("disabled index (col)"), index (col) #2=1 ("index (col)")) -> (element #1=w1139:dbl[], element #2=w1138:dbl[])  [unwired: 2 in]
          n399 = Divide(x=w1204, y=10.0) -> (x/y=w1202:dbl)
          n400 = Divide(x=w1199, y=10.0) -> (x/y=w1197:dbl)
          n401 = Divide(x=w1194, y=20.0) -> (x/y=w1192:dbl)
          n402 = Index Array(array=w1144, index (col) #1=0 ("disabled index (col)"), index (col) #2=1 ("index (col)")) -> (element #1=w1148:dbl[], element #2=w1147:dbl[])  [unwired: 2 in]
          n403 = global read "GVZeitenZyklen.vi" "ZyklusNummernGesamt"() -> (→"ZyklusNummernGesamt":i32[])
          n404 = local read "veränderte Methode benutzen"() -> (w1221:bool)
          n405 = Or(x=w1222, y=w1223) -> (x .or. y?=w1225:bool)
          n406 = Index Array(array=w1109, index (col) #1=0 ("disabled index (col)"), index (col) #2=1 ("index (col)")) -> (element #1=w1113:dbl[], element #2=w1112:dbl[])  [unwired: 2 in]
          n407 = Greater Or Equal?(x=w1108, y=w1113) -> (x >= y?=w1111:bool[])
          n408 = Less Or Equal?(x=w1108, y=w1112) -> (x <= y?=w1110:bool[])
          n409 = global read "GVZeitenZyklen.vi" "Big Ben, Methodenzeit, Zykluszeit0, Zykluszeit1, Zykluszeit2A, Zykluszeit2B"() -> (w1171:dbl[])
          n410 = Or(x=w1225, y=w1221) -> (x .or. y?=w1224:bool)
          n411 = And(x=w1111, y=w1110) -> (x .and. y?=→"MVOK?":bool[])
          n412 = Index Array(array=w1126, index (col) #1=0 ("disabled index (col)"), index (col) #2=1 ("index (col)")) -> (element #1=w1130:dbl[], element #2=w1129:dbl[])  [unwired: 2 in]
          n413 = global read "GVHK1Hz.vi" "Mod1Mod2Mod3/AITrapsMachs1Hz"() -> (w1104:dbl[])
          n414 = Array Subset(array=w1104, index=0 ("Index"), length=32 ("Länge")) -> (w1155:dbl[])
          "AIs1" <- w1155
          n415 = Greater Or Equal?(x=w1155, y=w1156) -> (x >= y?=w1153:bool[])
          n416 = Less Or Equal?(x=w1155, y=w1154) -> (x <= y?=w1152:bool[])
          n417 = And(x=w1153, y=w1152) -> (x .and. y?=→"AIs1OK?":bool[])
          n418 = Array Subset(array=w1104, index=32 ("Index"), length=32 ("Länge")) -> (w1143:dbl[])
          "AIs2" <- w1143
          n419 = Greater Or Equal?(x=w1143, y=w1148) -> (x >= y?=w1146:bool[])
          n420 = Less Or Equal?(x=w1143, y=w1147) -> (x <= y?=w1145:bool[])
          n421 = And(x=w1146, y=w1145) -> (x .and. y?=→"AIs2OK?":bool[])
          n422 = Array Subset(array=w1104, index=64 ("Index"), length=32 ("Länge")) -> (w1134:dbl[])
          "AIs3" <- w1134
          n423 = Greater Or Equal?(x=w1134, y=w1139) -> (x >= y?=w1137:bool[])
          n424 = Less Or Equal?(x=w1134, y=w1138) -> (x <= y?=w1136:bool[])
          n425 = And(x=w1137, y=w1136) -> (x .and. y?=→"AIs3OK?":bool[])
          n426 = Array Subset(array=w1104, index=96 ("Index"), length=6 ("Länge")) -> (w1103:dbl[])
          "schnelle Heizungen" <- w1103
          n427 = Greater Or Equal?(x=w1103, y=w1130) -> (x >= y?=w1128:bool[])
          n428 = Less Or Equal?(x=w1103, y=w1129) -> (x <= y?=w1127:bool[])
          n429 = And(x=w1128, y=w1127) -> (x .and. y?=→"SHOK?":bool[])
          n430 = To Long Integer(number=w1171) -> (32bit integer=→"Big Ben, Methodenzeit, Zykluszeit0, Zykluszeit1, Zykluszeit2A, Zykluszeit2B":i32[])
          n431 = Equal?(x=w1184, y=w1183) -> (x = y?=w1182:bool)
          n432 = call "AnzeigeGV.vi"("veränderte Methode benutzen"=w1221, "Zykluslängen [s]"=w1188, "Cluster1"=w1220, "Big Ben, Methodenzeit, Zykluszeit0, Zykluszeit1, Zykluszeit2A, Zykluszeit2B"=w1171, "Zyklusnummern 0, 1, 2A, 2B"=w1191, "Cluster2"=w1219, "AnzeigeEinstellungen"=w1218, "dargestellte Größe 1"="dargestellte Größe 1", "Zeitachse1"="Zeitachse1", "dargestellte Größe 2"="dargestellte Größe 2", "Zeitachse2"="Zeitachse2") -> ("Anzeige2"=→"Housekeeping2":cluster{dbl[], dbl[]}, "Cluster1"=w1213:cluster{dbl[], dbl[], dbl[], dbl[]}, "x1Inkr"=w1208:dbl, "Cluster2"=w1212:cluster{dbl[], dbl[], dbl[], dbl[]}, "Anzeige1"=→"Housekeeping1":cluster{dbl[], dbl[]}, "AnzeigeEinstellungen"=w1210:T17, "x2Max"=w1172:dbl, "x2Inkr"=w1207:dbl, "x1Max"=w1173:dbl)  [unwired: 8 in]
          n433 = Divide(x=w1186, y=20.0) -> (x/y=w1187:dbl)
          n434 = Select(t=w1180, s=w1182, f=w1181) -> (s? t:f=w1175:cluster{dbl[], dbl[]})
          n435 = property on="Housekeeping1" class="XYGraph (strict)"("XScale.Minimum"=w1189, "XScale.Maximum"=w1173, "XScale.Increment"=w1208, "YScale.Minimum"="HK1YMin", "YScale.Maximum"="HK1YMax", "YScale.Increment"=w1202) -> ()  [unwired: 2 in, 2 out]
          n436 = property on="Housekeeping2" class="XYGraph (strict)"("XScale.Minimum"=w1189, "XScale.Maximum"=w1172, "XScale.Increment"=w1207, "YScale.Minimum"="HK2YMin", "YScale.Maximum"="HK2YMax", "YScale.Increment"=w1197) -> ()  [unwired: 2 in, 2 out]
          n437 = property on="Detektor 2" class="XYGraph (strict)"("XScale.Minimum"=w1189, "XScale.Maximum"=w1186, "XScale.Increment"=w1187, "YScale.Minimum"="DetYMin", "YScale.Maximum"="DetYMax", "YScale.Increment"=w1192) -> ()  [unwired: 2 in, 2 out]
          n438 = Select(t=w1175, s=w1176, f=cluster{dbl[], dbl[]} {[], []} ("s? t:f")) -> (s? t:f=w1168:cluster{dbl[], dbl[]})
          n439 = Build Array(w1179, w1168) -> (→"Detektor 2":cluster{dbl[], "ECD2Chrom":dbl[]}[])
        }
        n440 = global read "GVZeitenZyklen.vi" "Big Ben, Methodenzeit, Zykluszeit0, Zykluszeit1, Zykluszeit2A, Zykluszeit2B"() -> (w972:dbl[])
        n441 = Index Array(array=w972, index=3 ("Index")) -> (element=w970:dbl)
        n442 = while {
          tunnel: w1014 -> [w1041]
          tunnel: w1013 -> [w1040]
          tunnel: w935 -> [w1055]
          shift-right: [w1056] -> w1007
          shift-left: w1012 -> [w1057]
          tunnel: w932 -> [w1051]
          tunnel: w931 -> [w1045]
          shift-right: [w1042] -> _
          shift-left: w970 -> [w1046]
          stop <- w1058 stop-if-true
          n443 = Less?(x=w1046, y=w1051) -> (x < y?=w1049:bool)
          n444 = Less?(x=w1046, y=w1045) -> (x < y?=w1047:bool)
          n445 = call "Bis zum nächsten Vielfachen warten13"("Count(mSec)"=u32 100 ("Zu wartende ms")) -> ()  [unwired: 1 out]
          n446 = global read "GVMethodenwechsel.vi" "Methodenwechsel?"() -> (w1060:bool)
          n447 = global read "gvbooleschRT.vi" "global stop RT"() -> (w1061:bool)
          n448 = local read "veränderte Methode benutzen"() -> (w1059:bool)
          n449 = global read "GVZeitenZyklen.vi" "Big Ben, Methodenzeit, Zykluszeit0, Zykluszeit1, Zykluszeit2A, Zykluszeit2B"() -> (w1053:dbl[])
          n450 = Compound Arithmetic op=OR(w1061, w1060, w1059) -> (w1058:bool)
          n451 = Index Array(array=w1053, index=3 ("Index")) -> (element=w1042:dbl)
          n452 = Greater Or Equal?(x=w1042, y=w1051) -> (x >= y?=w1050:bool)
          n453 = Greater Or Equal?(x=w1042, y=w1045) -> (x >= y?=w1048:bool)
          n454 = And(x=w1048, y=w1047) -> (x .and. y?=w1044:bool)
          n455 = And(x=w1050, y=w1049) -> (x .and. y?=w1039:bool)
          n456 = Or(x=w1039, y=w1044) -> (x .or. y?=w1043:bool)
          n457 = And(x=w1055, y=w1043) -> (x .and. y?=w1054:bool)
          n458 = case shown="True" w1054 {
            tunnel: w1057 -> [w1063 w1064]
            tunnel: [w1063 w1068] -> w1056
            tunnel: w1041 -> [_ w1067]
            tunnel: w1040 -> [_ w1066]
            tunnel: w1039 -> [_ w1065]
            frame False {
            }
            frame True {
              n459 = call "MSDateienSchicken12-15.vi"("MSNummer"=w1064, "MSa?"=w1065, "Dateipfad:fromcriordy"=w1066, "Dateipfad:fromcriocmd"=w1067) -> ()  [unwired: 1 in]
              n460 = Increment(x=w1064) -> (x+1=w1068:i32)
            }
          }
        }
      }
      n461 = Add Array Elements(numeric array=w486) -> (sum=w496:i32)
      n462 = Index Array(array=w486, index #1=0 ("Index"), index #2=1 ("Index")) -> (element #1=w507:i32, element #2=w505:i32)
      n463 = Split 1D Array(array=w485, index=w507) -> (first subarray=w511:dbl[], second subarray=w515:dbl[])
      n464 = Split 1D Array(array=w483, index=w507) -> (first subarray=w514:string[], second subarray=w516:string[])
      n465 = Split 1D Array(array=w484, index=w507) -> (first subarray=w504:string[], second subarray=w506:string[])
      n466 = Initialize Array(-1.0 ("Element"), w496) -> (w481:dbl[])
      n467 = Split 1D Array(array=w516, index=w505) -> (first subarray=w513:string[], second subarray=w512:string[])
      n468 = Split 1D Array(array=w515, index=w505) -> (first subarray=w510:dbl[], second subarray=w509:dbl[])
      n469 = Split 1D Array(array=w506, index=w505) -> (first subarray=w503:string[], second subarray=w502:string[])
      n470 = Bundle(w514, w513, w512, w511, w510, w509) -> (w508:T28)  [unwired: 1 in]
      n471 = Bundle(w504, w503, w502) -> (w501:cluster{string[], string[], string[]})  [unwired: 1 in]
      n472 = Initialize Array(0.0, 8 ("Dimension")) -> (w431:dbl[])
      n473 = Bundle(w500, w500, w500) -> (w499:cluster{i32, i32, i32})  [unwired: 1 in]
      n474 = Initialize Array("x", 8 ("Dimension")) -> (w436:string[])
      n475 = case shown="True" TRUE ("SerielleKomm.") {
        tunnel: bool[] [TRUE, TRUE, TRUE, TRUE, TRUE, TRUE, TRUE, TRUE] -> [_ w573]
        tunnel: w436 -> [_ w572]
        tunnel: w508 -> [_ w571]
        tunnel: w507 -> [_ w570]
        tunnel: w505 -> [_ w569]
        tunnel: w501 -> [_ w568]
        tunnel: w499 -> [_ w567]
        tunnel: w498 -> [_ w566]
        tunnel: w485 -> [_ w565]
        tunnel: w482 -> [_ w564]
        tunnel: w481 -> [_ w563]
        tunnel: w480 -> [_ w560]
        tunnel: w459 -> [_ w562]
        tunnel: w431 -> [_ w561]
        tunnel: w430 -> [_ w559]
        frame False {
        }
        frame True {
          n476 = while {
            tunnel: w560 -> [w584]
            tunnel: w559 -> [w577]
            shift-right: [w576] -> _
            shift-left: errorcluster {"status"=FALSE, "code"=0, "source"=""} ("error out") -> [w575]
            stop <- w586 stop-if-true
            n477 = String To Byte Array(string=w577) -> (unsigned byte array=w580:u8[])
            n478 = call "Warten6"("Count(mSec)"=u32 500) -> ()  [unwired: 1 out]
            n479 = Join Numbers(hi=w580, lo=u8 5) -> ((hi.lo)=w582:u16[])
            n480 = Join Numbers(hi=w580, lo=u8 6) -> ((hi.lo)=w578:u16[])
            n481 = xnode "Invoke Method"("FPGA VI Reference In"=w584, "error in"=w575, "Data"=w582) -> ("FPGA VI Reference Out"=w581:refnum<k20>, "error out"=w574:errorcluster)  [unwired: 1 in, 1 out]
            n482 = xnode "Invoke Method"("FPGA VI Reference In"=w581, "error in"=w574, "Data"=w578) -> ("error out"=w576:errorcluster)  [unwired: 1 in, 2 out]
            "FIFOwriteRS485" <- w576
            n483 = global read "gvbooleschRT.vi" "global stop RT"() -> (w586:bool)
          }
          n484 = while {
            shift-right: [w724] -> _
            shift-left: w573 -> [w739]
            shift-right: [w743] -> _
            shift-left: w563 -> [w749]
            tunnel: w560 -> [w738]
            shift-right: [w725] -> _
            shift-left: w572 -> [w727]
            tunnel: w564 -> [w729]
            tunnel: w565 -> [w726]
            shift-right: [w730] -> _
            shift-left: w566 -> [w745]
            tunnel: w570 -> [w747]
            tunnel: w569 -> [w748]
            tunnel: w571 -> [w750]
            tunnel: w568 -> [w732]
            shift-right: [w731] -> _
            shift-left: w567 -> [w733]
            shift-right: [w736] -> _
            shift-left: w562 -> [w737]
            shift-right: [w740] -> _
            shift-left: w561 -> [w741]
            shift-right: [w721] -> _
            shift-left: errorcluster {"status"=FALSE, "code"=0, "source"=""} ("error out") -> [w720]
            stop <- w744 stop-if-true
            n485 = for {
              tunnel: w739 -> [w754] mode=indexing
              tunnel: w741 -> [w751] mode=indexing
              tunnel: [w758] -> w740 mode=indexing
              tunnel: [w755] -> w734 mode=indexing
              n486 = global read "GVZeitenZyklen.vi" "Big Ben, Methodenzeit, Zykluszeit0, Zykluszeit1, Zykluszeit2A, Zykluszeit2B"() -> (w761:dbl[])
              n487 = Index Array(array=w761, index=0 ("Index")) -> (element=w759:dbl)
              n488 = Subtract(x=w759, y=w751) -> (x-y=w757:dbl)
              n489 = Greater?(x=w757, y=0.1) -> (0:w753:bool)
              n490 = Or(x=w754, y=w753) -> (x .or. y?=w752:bool)
              n491 = Select(t=w753, s=w753, f=w754) -> (s? t:f=w755:bool)
              n492 = Select(t=w759, s=w752, f=w751) -> (s? t:f=w758:dbl)
            }
            n493 = global read "GVHorstSP.vi" "HorstSP"() -> (w743:dbl[])
            n494 = Not Equal?(x=w743, y=w749) -> (x != y?=w746:bool)
            n495 = call "NeueSP.vi"("Anzahl2"=w748, "Anzahl1"=w747, "AlteSP"=w749, 7:"NeueSP"=w743, "BefehleCluster"=w745, 10:"NeueSP"=w746, "ClusterFest"=w750) -> ("BefehleCluster"=w735:T29)  [unwired: 4 in]
            n496 = call "Warten3"("Count(mSec)"=u32 50) -> ()  [unwired: 1 out]
            n497 = call "MPVSenden-01-17.vi"("Ventilposition"=w737, "error in"=w720, "FPGA VI Reference In"=w738) -> ("Ventilposition"=w736:i32, "error out"=w723:errorcluster, "FPGA VI Reference Out"=w719:refnum<k20>)
            n498 = call "Senden-01-17.vi"("error in"=w723, "BefehlsCluster"=w735, "AbfragenCluster"=w732, "Abfragenr.Cluster"=w733, "Senden?"=w734, "FPGA VI Reference In"=w719) -> ("BefehlsCluster"=w730:T29, "error out"=w722:errorcluster, "Senden?"=w728:bool[], "Abfragenr.Cluster"=w731:cluster{i32, i32, i32})  [unwired: 1 in]
            n499 = call "SeriellRead-01-17.vi"("SkalierungsfaktorHorst"=w726, "VorwortHorst"=w729, "error in"=w722, "Zwischenspeicher"=w727, "Senden?"=w728, "FPGA VI Reference In"=w719) -> ("Senden?"=w724:bool[], "Zwischenspeicher"=w725:string[], "error out"=w721:errorcluster)  [unwired: 3 in]
            "SerielleKomm." <- w721
            n500 = global read "gvbooleschRT.vi" "global stop RT"() -> (w744:bool)
          }
        }
      }
      n501 = flat-sequence {
        frame #0 {
          n502 = global write "Emulate Licor output GV.vi" "Emulator an?"(FALSE ("Emulator an?")) -> ()
        }
        frame #1 {
          n503 = control-ref of="GUI_Cluster_Parameter"() -> (w529:refnum<vi>)
          n504 = control-ref of="GUI_Cluster_Graph"() -> (w530:refnum<vi>)
          n505 = control-ref of="GUI_Cluster_sdv"() -> (w528:refnum<vi>)
          n506 = call "licore (main).vi"("GUI_Cluster_Graph (extern)"=w530, "GUI_Cluster_Parameter (extern)"=w529, "GUI_Cluster_sdv (extern)"=w528) -> ()  [unwired: 13 in]
        }
      }
    }
    frame #2 {
      n507 = xnode "Read/Write Control"("FPGA VI Reference In"=w1351, "global stop"=TRUE) -> ("FPGA VI Reference Out"=w1350:refnum<k20>)  [unwired: 1 in, 1 out]
      n508 = xnode "Close FPGA VI Reference"("FPGA VI Reference In"=w1350) -> ()  [unwired: 1 in, 1 out]
    }
    frame #3 {
    }
    frame #4 {
    }
  }
